vi "Main7.vi"() -> ()   [LabVIEW 2017]
uses:
  <vilib>/Analysis/2dsp.llb/Real FFT.vi
  <vilib>/Analysis/NI_AALPro.lvlib
  atmcd32d.dll
panel:
  in  "index (row)":i32
  out "Angle Integrated Spectrum 2":T1(graph)
  in  "Area Parameteres":T2={"Center angle (deg)"=90.0, "Arc length (deg)"=90.0, "Angle step (deg)"=10.0, "Outer radius "=0.7640449438202247, "Inner radius "=0.0, "Radius"=0.0, "Radial step "=0.5}
  in  "Tab Control":T3(tab)
  out "Current angle":dbl
  in  "Exposure time [ms]":u32=100
  out "Count":i32
  in  "Integration time [s]":dbl=1.0
  out "Ready":bool
  out "Connected":bool
  out "Device":refnum<visa-resource-name>
  in  "Exit":bool
  in  "Take image":bool
  in  "Spectrum":T4(tab)
  out "Fully Integrated Spectrum":dbl(graph)
  out "Angular distribution":dbl[][](graph)
  out "Angle Integrated Spectrum":T5(graph)
  out "Angular distribution 2":dbl[][](graph)
  in  "Energy/Radius":enum32{"Radius", "Energy"}(radio)
  out "Spectrogram up":dbl[][](graph)=[[0.0010313840536425023, 0.0010313840536425023, 0.0010274759814052766, 0.0010401531177745159, 0.00104452387932524, 0.0010522711712232782, 0.001047206375702307, 0.0010453914217880493, 0.0010393489196820073, 0.0010272942106035452, 0.0010408196107141979, 0.0010468510964080136, 0.001062026204249532, 0.001106433361933133, 0.001154520001300267, 0.0011934960677563772, 0.001214033414248973, 0.0012241024150236718, 0.0012391453259184763, 0.0012555680424446059, 0.0012925281054633312, 0.001352528994653044, 0.0014089853532089937, 0.0014660421062312687, 0.0015363130457188075, 0.0015691474623588406, 0.0016108363203256395, 0.0016140062929437132, 0.0015863330654316305, 0.001566139981821102, 0.0015480455247396548, 0.0015630250912641588, 0.0016089194645982896, 0.0016388896140595243, 0.0016752961023638853, 0.001688323009821305, 0.0016919033437948032, 0.0017147706614732288, 0.0017464097973867246, 0.001779717919752482, 0.001837171263614898, 0.00188523587015758, 0.001909243386501412, 0.0019293676175355272, 0.0019505631946586353, 0.0019533283141273984, 0.001977616748982997, 0.0019911972311547808, 0.002017708227177005, 0.002053718124641225, 0.0020883013967221585, 0.002112669700566397, 0.0021315656016372966, 0.0021208218456137463, 0.002105299720787104, 0.002099830072116822, 0.0021012126318512036, 0.0020908214010188896, 0.002095054457416787, 0.002100080695494967, 0.0021084586769929523, 0.0020993728910094368, 0.002104955457905037, 0.0020792872174181134, 0.0020928346503532183, 0.0020942117018814864, 0.002102964241395161, 0.0021093372358679877, 0.002121036665652156, 0.002136567052787968, 0.002154127213876447, 0.002169360157882152, 0.0021869395976920275, 0.0021825908689657556, 0.002171045668952753, 0.0021674267775364637, 0.0021489908116760054, 0.002157660728097984, 0.002145658346977596, 0.002135917084466625, 0.00209696855904108, 0.0020850653256307278, 0.0020535996982097935, 0.002049595232365589, 0.0020524236962046524, 0.0020767176392663643, 0.002111884781195284, 0.002137809153266466, 0.0021668842192343256, 0.00216397037820051, 0.0021656008072099796, 0.0021352698702483386, 0.0021013916485498785, 0.0020823029602650214, 0.0020479290000163844, 0.0020333460243320213, 0.0020002169186649392, 0.0019659586307446764, 0.0019358700548520106, 0.0019274369912928948, 0.0019173046461478957, 0.001900014387158957, 0.0018599917615413628, 0.001814549061108504, 0.0017608991335671654, 0.0017321325271416374, 0.0017011240808280886, 0.0016809695546603515, 0.0016804848325224012, 0.001677022924980334, 0.0016912533754734602, 0.0016999535870290603, 0.0017145172839920274, 0.001701024933118053, 0.0017087557003977521, 0.0017038864461937952, 0.0017154509249281934, 0.0017378638156022909, 0.001773105318313737, 0.0017971238510697952, 0.001824766783448256, 0.0018273914436611356, 0.0018233456662710829, 0.001811169776658133, 0.001808649772361402, 0.0017980740166243004, 0.0017838545825434003, 0.001763256645783561, 0.0017210445082360198, 0.001701132343137258, 0.0016754062664861471, 0.001664623953019805, 0.0016487024832499652, 0.0016273141189128994, 0.0016010950578146683, 0.0015728930425157306, 0.0015352912734848325, 0.0015149109108664593, 0.001483448037548582, 0.0014523514599372237, 0.0014315579818603703, 0.0014274984339550348, 0.0014181675327994876, 0.0014143999198181453, 0.0014053113797315735, 0.0013993515007172275, 0.001408693418285001, 0.0013985390403155494, 0.001397974449188959, 0.0013917694550025816, 0.0013787315311329358, 0.0013626448151797038, 0.0013449083914956062, 0.0013370509354753064, 0.001325880293477993, 0.0013185543793476045, 0.001294420174263172, 0.00127875483607759, 0.0012659041912157889, 0.0012433398248735822, 0.001228894554342046, 0.0012003400138518715, 0.001183988904005212, 0.0011747543964566436, 0.0011585547622780935, 0.0011605046672421217, 0.0011473565792502146, 0.0011370039058606926, 0.0011340652778993677, 0.0011226770617605876, 0.0011216442731143861, 0.0011107600578349525, 0.0011026409620242816, 0.0010866919512238764, 0.0010731362559796018, 0.001051089661012024, 0.0010301832647098524, 0.001009888279286232, 0.0009965887156262153, 0.0009909235256389188, 0.0009767536654130364, 0.0009747817276245561, 0.0009568910741692924, 0.000949947980363763, 0.000956703795161448, 0.0009593917997446279, 0.0009746082191319944, 0.0009815127554947322, 0.0009862085012061277, 0.0009848589907084247, 0.0009587748806599638, 0.0009397330121270677, 0.0009244532483694009, 0.0009160174307072283, 0.0009138141482619988, 0.0009141501488348964, 0.0009184162544694721, 0.0009130457535092251, 0.000912208506180038, 0.0009004897976744733, 0.0008954966088329721, 0.000888658170943591, 0.000878327530378521, 0.0008779392018475493, 0.0008724833236925496, 0.0008753007711193868, 0.0008733894235981503, 0.0008842763929806406, 0.0008803270091975667, 0.0008834474079606231, 0.0008812331091031674, 0.0008784927765619131, 0.0008838109495640858, 0.0008909550928927427, 0.000899184352825675, 0.0009081654828930417, 0.000914194214483801, 0.0009259542345352136, 0.0009387635678511666, 0.0009425339349355657, 0.0009425063939050002, 0.0009326494590656548, 0.0009267529244216092, 0.0009192645182108854, 0.0009126023429171226, 0.0009054058716303917, 0.0008956756255316468, 0.0008975015958581308, 0.0008902445343041561, 0.0008840973762819658, 0.0008824283898297043, 0.0008799772381093866, 0.000884678492026895, 0.0008933897199947213, 0.0008983829088362226, 0.000893860671617389, 0.0008973749071175302, 0.0009013435696219998, 0.0009055848883290665, 0.0009138995254567515, 0.0009202174378684471, 0.000930589389979365, 0.000922150818214136, 0.0009280666315795773, 0.0009267253833910438, 0.0009243623629685353, 0.0009317653919845064, 0.0009418922289233926, 0.0009494384712983037, 0.0009643051195974898, 0.0009718458537662879, 0.0009862966325039368, 0.0009917001827008621, 0.0009979795376697665, 0.001014038712592433, 0.0010172830459930335, 0.0010330585483008768, 0.0010469640146333317, 0.001060098332109956, 0.0010826544361429932, 0.0011030761103072145, 0.0011350760337211167, 0.0011531154087414334, 0.0011576624328877758, 0.0011768364983673857, 0.0011841624124977737, 0.0011999406689086737, 0.0012165093528967996, 0.0012281895039595726, 0.0012561601746017613, 0.0012707651831105765, 0.001307240523991351, 0.001333627585376031, 0.0013666217399933432, 0.0014024911782016796, 0.0014332324765187446, 0.0014678102403935655, 0.0014988241949132272, 0.0015329365153714935, 0.0015343879276822883, 0.0015720971067323913, 0.0016118636007657278, 0.001651087536496926, 0.0016970920739533186, 0.001745473402347502, 0.0017665615694514051, 0.0018051024876245825, 0.0018256783915599696, 0.0018815618966801597, 0.0018972630382054765, 0.0019475088943689358, 0.001967589059754146, 0.0019944801219981727, 0.0020293085092511383, 0.0020797967264835726, 0.002127649267090901, 0.002177592171918141, 0.002209096356781867, 0.0022576126362258207, 0.0022860239633570555, 0.002367479315357191, 0.00239798651491445, 0.002459918030346795, 0.002492961758819125, 0.0025305745442622493, 0.0025619850896220525, 0.0025918974029190997, 0.0026126908809959533, 0.0026649499864937407, 0.002671884817990101, 0.0027487573425041584, 0.0027664331759210126, 0.0028080311484869457, 0.002835572179052315, 0.002897776350687257, 0.0029281981730497637, 0.0029626547563900967, 0.002993387792397992, 0.0030170785868903222, 0.0030149964849795806, 0.0030319039236436605, 0.0030360240618162396, 0.0030334957952103388, 0.0030378693108641195, 0.003026379192912247, 0.0030242502712495446, 0.0030348563221202682, 0.0030418489897808152, 0.0030719182869520852, 0.0030982750532031434, 0.0030908086798168716, 0.0031010319103627363, 0.0031036813575031253, 0.0030762670156783568, 0.003066933360419753, 0.003042223547796504, 0.0030263378813663996, 0.003004663090311454, 0.0029920548065186284, 0.0029706664421815625, 0.0029578268137319874, 0.0029413352446294445, 0.0029132489016588815, 0.0028961762168114094, 0.002857943758180564, 0.00283680050901553, 0.0028030104186148787, 0.0027938640423641197, 0.0027516161014768444, 0.002719478472910115, 0.0026733913123620267, 0.002627637398283779, 0.0025728335015617514, 0.0025436510255746865, 0.002504355483164018, 0.0024615594757684913, 0.002436053727361903, 0.0024182842544411267, 0.0024007185851465346, 0.0023905779776923655, 0.0023550968680150007, 0.002333292634116398, 0.002292746728918062, 0.0022553735504408563, 0.0022384468330553806, 0.002203128215458351, 0.00217902430550754, 0.002143711196116624, 0.0021122262899742946, 0.0020506142504965077, 0.00203825383597877, 0.0020262487007553258, 0.0020074629638066875, 0.0019932738248594093, 0.0019544327094530695, 0.0019488088310116213, 0.0019049882972790627, 0.0018915620448784454, 0.0018528393559035367, 0.001821197465886984, 0.0017890212798774634, 0.0017354539754278208, 0.0016897689139259869, 0.001663423164087155, 0.0016456371665480398, 0.0016412085688331283, 0.001628644350689207, 0.0016130809143167168, 0.0016073331012377244, 0.001603339651805746, 0.0015941712427305346, 0.001588935692820058, 0.0015824029603699523, 0.00157714813173808, 0.0015643332902160138, 0.0015630746651191763, 0.0015527274999357675, 0.0015555421932595482, 0.0015637163711313498, 0.0015732180266764021, 0.001592557338339404, 0.001584653062567143, 0.0015960522951181493, 0.0016165015103129358, 0.0016268707083207973, 0.0016398039762742945, 0.001641899848700319, 0.0016484215647381982, 0.0016487190078683044, 0.0016555629539637985, 0.0016557612493838694, 0.0016741145921526312, 0.0017004658501975761, 0.0017330110860166727, 0.0017605190673453631, 0.0017664348807108045, 0.0017779084740443371, 0.001790398331405732, 0.0018131775177863488, 0.0018366452299310996, 0.0018605453362557267, 0.0018882543671075445, 0.0018984252696953353, 0.001914192509694009, 0.0019416316384462862, 0.0019781785860065308, 0.0020108477564631713, 0.0020298097560074277, 0.0020661143424986973, 0.002068810609391047, 0.002110609631480107, 0.002115869968318093, 0.0021256800834054774, 0.0021556667574850513, 0.002178443189762611, 0.0021840174943490416, 0.002213334921385877, 0.002212183706308245, 0.00223874152208243, 0.0022391546375409104, 0.002258397555596934, 0.0022739802706908193, 0.0023094503639559585, 0.002319709397841558, 0.002351866305129683, 0.002368812301236555, 0.0023749456887434623, 0.002389630566240917, 0.0023986777947816403, 0.00241149814450982, 0.0024190003212358263, 0.0024229882624616918, 0.002422095933071374, 0.002423731870286957, 0.0024201625527256847, 0.0024417767535133868, 0.0024415812121963724, 0.002455808908586442, 0.002457513698378438, 0.0024465385976981386, 0.0024522313287160006, 0.0024169705472831585, 0.0024148361174143426, 0.0023995701241719585, 0.0023793853028705996, 0.0023548297200185167, 0.002332361747283289, 0.0023205108418310103, 0.0022940521737668603, 0.0022523164960481005, 0.0022274744864781374, 0.0022039158889325208, 0.0021684926154193433, 0.0021411526343771015, 0.002118635087786856, 0.002083801192327777, 0.002047124801923875, 0.0020278653592495127, 0.0019697703093749233, 0.0019519264756716211, 0.0019212622922401392, 0.0018812286502103187, 0.0018427428140982722, 0.001812265909674635, 0.00175640994558501, 0.0017214080498394828, 0.0016736711815605288, 0.0016349457384825634, 0.0015946835058990505, 0.0015675610989982752, 0.0015259052902681545, 0.0014996366553149056, 0.001476708747369236, 0.001439175830914751, 0.0014011692087345419, 0.0013630882257718063, 0.0013162216540587178, 0.0012905451512626243, 0.0012539458757443056, 0.0012235736272368167, 0.0012001196856073486, 0.001185272316029558, 0.0011544346241055146, 0.0011379100057662933, 0.0010844501113358553, 0.0010647610285846733, 0.0010130802847287583, 0.0009929670701068693, 0.0009656849252288149, 0.0009476042386626501, 0.0009280005331062204, 0.0009123489654359212, 0.0008921173243826012, 0.0008740696870531149, 0.000861342976828858, 0.0008399518583887359, 0.0008269304591374295, 0.000805963472568014, 0.0007840931401960546, 0.0007730684656607372, 0.0007618757908389714, 0.000755502796366145, 0.0007484440302322409, 0.0007361304354664644, 0.0007236515945172958, 0.0007035631668229157, 0.0006909796699575985, 0.0006775396470416985, 0.0006603843391025302, 0.0006506954045496334, 0.0006404831904159946, 0.0006315406177914192, 0.000626814576946402, 0.0006201799426832045, 0.0006156053775062967, 0.0006078663479174281, 0.0005998298751984535, 0.0005900335306263518, 0.0005812644664943382, 0.0005748804556092857, 0.0005698349388097101, 0.000566761359798615, 0.0005616442363195694, 0.0005622749259195163, 0.0005532993040582626, 0.0005422911541412846, 0.0005348495676825219, 0.0005325361211150309, 0.0005320376284617976, 0.0005307018884793774, 0.0005264054877111798, 0.0005264054877111798, 0.0005228637111804734, 0.0005181238998201733, 0.0005176309153730532, 0.0005136154331166225, 0.0005124091359778592, 0.0005101562796776121, 0.0005055431570579128, 0.0004995529829099451, 0.0004920150028442035, 0.0004884759804165536, 0.00048560345092858563, 0.000481450263519328, 0.000479029406932632, 0.00047415189041950524, 0.00047243608421528277, 0.0004715299843096821, 0.00047353772543789753, 0.00047000971942247376, 0.0004698554896513077, 0.0004721276246729506, 0.0004682388311571205, 0.0004696351614067847, 0.0004644106279085342, 0.00046173088563452376, 0.0004594807834373332, 0.0004550053659704607, 0.0004509155229315034, 0.00044808430498938354, 0.0004430277717775818, 0.0004410696045043841, 0.00043787759906185783, 0.00043347929648056836, 0.0004299017166101269, 0.00042542354504019795, 0.00042215993291820175, 0.00041868425486085215, 0.000416883071461877, 0.0004110388647759057, 0.0004118981449295452, 0.00040788541677617095, 0.00040867033614728403, 0.00040761000647051725, 0.0004041866563712419, 0.00040178507850594175, 0.00039903372955246133, 0.0003977007436730975, 0.0003977310388067194, 0.00039884645054461687, 0.00039690480788975835, 0.000394671230310907, 0.0003933712936682215, 0.00039117076532604856, 0.0003899947633209073, 0.00038895095826247983, 0.00038990112381698505, 0.00038822662915861066, 0.0003852577060636639, 0.00038354740806555447, 0.0003831673418437523, 0.00038108523993301045, 0.00038199133983861106, 0.0003807712721845652, 0.0003789921216100424, 0.0003772350038599718, 0.00037759028315426514, 0.0003756155912627282, 0.0003736216206497954, 0.000373136898511845, 0.0003710079768491419, 0.0003707132878220925, 0.0003699917128212798, 0.00036924259678990177, 0.0003697686304737003, 0.000369484957858877, 0.0003692976788510325, 0.00037006056539769325, 0.00036974108944313496, 0.00036845492331573224, 0.0003671825277036122, 0.0003674441674939832, 0.00036729820003198675, 0.00036671708428705744, 0.0003670723635813507, 0.0003662516408705027, 0.0003653593114801848, 0.0003654336722627113, 0.00036621859163382426, 0.0003649076385789127, 0.0003645000313265452, 0.00036404009611610357, 0.00036481399907499045, 0.00036354435756592694, 0.0003624454704463687, 0.00036318632416857717, 0.000362616224835874, 0.00036201858447260554, 0.0003629026515537539, 0.00036316429134412485, 0.0003618092726403087, 0.00036178173160974337, 0.0003609059268377646, 0.0003606580575626763, 0.00035972441662651027, 0.00035978776099681063, 0.0003598290725426587, 0.0003593278257863689, 0.00035902487445014993, 0.0003587962838964574, 0.00035836939792269413, 0.00035583837721373673, 0.0003554059830338604, 0.0003547532606094612, 0.0003549102444836838, 0.00035429057129596295, 0.0003543126041204152, 0.0003549185067928534, 0.0003548248672889311, 0.00035513057272820676, 0.0003544998831282598, 0.00035434014515098067, 0.000354516407746599, 0.00035333489753534467, 0.0003535855209134895, 0.0003530154215807864, 0.0003527152243476239, 0.0003532798154742139, 0.00035263260125592777, 0.0003519964034498677, 0.000351608074918896, 0.00035093882787615757, 0.000349443349916458, 0.00034942957940117537, 0.0003491624314046913, 0.00034956453045094566, 0.00034901095573658175, 0.00034910184113744744, 0.0003489310867479422, 0.0003488181685226241, 0.0003479836752964935, 0.0003476917403725006, 0.00034843259409470895, 0.0003489586277785075, 0.0003480910853156984, 0.0003474548875096384, 0.0003469619030625183, 0.00034665344352018617, 0.0003463918037298151, 0.00034654052529486815, 0.00034605304905386115, 0.0003454196053508576, 0.00034516347376659963, 0.00034559862204953256, 0.0003448357355028718, 0.0003449403914190202, 0.00034430419361296017, 0.00034424635744877293, 0.000344852260121211, 0.0003448384896059283, 0.0003451028834993559, 0.0003437423565894266, 0.0003425580922751158, 0.00034259664971790727, 0.0003416354677511759, 0.00034174838597649394, 0.00034173461546121124, 0.0003417869434192854, 0.0003409965158420593, 0.00034094143378092864, 0.0003408477942770064, 0.0003402501539137379, 0.0003404980231888262, 0.0003398783500011054, 0.00033904936498108774, 0.00033842969179336696, 0.00033828372433137053, 0.0003380661501899041, 0.00033740791955939176, 0.000338358085113897, 0.0003377081167925543, 0.00033727847671573453, 0.000337388640837996, 0.00033701959102842003, 0.00033749605085720095, 0.00033774116602923275, 0.0003364384752834908, 0.000335931720321088, 0.0003357031297673954, 0.00033592070390886183, 0.0003353395881639325, 0.00033492922680850853, 0.00033513303043469225, 0.00033468961984258985, 0.0003348713906443213, 0.00033494024322073466, 0.0003348108003770775, 0.00033487689885043436, 0.00033441145543387964, 0.0003341993894985263, 0.0003345464064836499, 0.00033424896335354395, 0.00033390194636842026, 0.00033334837165405635, 0.00033337040447850867, 0.0003331583385431553, 0.0003329132233711235, 0.0003332326993256818, 0.0003335301424557878, 0.0003335026014252224, 0.00033401761869679484, 0.0003333428634479433, 0.00033282509207331433, 0.00033313630571870306, 0.0003330839777606288, 0.00033270666564188324, 0.00033214758272140626, 0.00033204843501137094, 0.00033124974512497527, 0.0003311781384455053, 0.00033189695934326144, 0.0003313213518044452, 0.0003320980088663886, 0.0003318336149729611, 0.00033207873014499283, 0.0003325304030462649, 0.0003314094831022544, 0.00033175650008737803]]
  out "Range scan":dbl[][](graph)
  out "Spectrogram down":dbl[][](graph)=[[0.0010313840536425023, 0.0010313840536425023, 0.0010274759814052766, 0.0010401531177745159, 0.00104452387932524, 0.0010522711712232782, 0.001047206375702307, 0.0010453914217880493, 0.0010393489196820073, 0.0010272942106035452, 0.0010408196107141979, 0.0010468510964080136, 0.001062026204249532, 0.001106433361933133, 0.001154520001300267, 0.0011934960677563772, 0.001214033414248973, 0.0012241024150236718, 0.0012391453259184763, 0.0012555680424446059, 0.0012925281054633312, 0.001352528994653044, 0.0014089853532089937, 0.0014660421062312687, 0.0015363130457188075, 0.0015691474623588406, 0.0016108363203256395, 0.0016140062929437132, 0.0015863330654316305, 0.001566139981821102, 0.0015480455247396548, 0.0015630250912641588, 0.0016089194645982896, 0.0016388896140595243, 0.0016752961023638853, 0.001688323009821305, 0.0016919033437948032, 0.0017147706614732288, 0.0017464097973867246, 0.001779717919752482, 0.001837171263614898, 0.00188523587015758, 0.001909243386501412, 0.0019293676175355272, 0.0019505631946586353, 0.0019533283141273984, 0.001977616748982997, 0.0019911972311547808, 0.002017708227177005, 0.002053718124641225, 0.0020883013967221585, 0.002112669700566397, 0.0021315656016372966, 0.0021208218456137463, 0.002105299720787104, 0.002099830072116822, 0.0021012126318512036, 0.0020908214010188896, 0.002095054457416787, 0.002100080695494967, 0.0021084586769929523, 0.0020993728910094368, 0.002104955457905037, 0.0020792872174181134, 0.0020928346503532183, 0.0020942117018814864, 0.002102964241395161, 0.0021093372358679877, 0.002121036665652156, 0.002136567052787968, 0.002154127213876447, 0.002169360157882152, 0.0021869395976920275, 0.0021825908689657556, 0.002171045668952753, 0.0021674267775364637, 0.0021489908116760054, 0.002157660728097984, 0.002145658346977596, 0.002135917084466625, 0.00209696855904108, 0.0020850653256307278, 0.0020535996982097935, 0.002049595232365589, 0.0020524236962046524, 0.0020767176392663643, 0.002111884781195284, 0.002137809153266466, 0.0021668842192343256, 0.00216397037820051, 0.0021656008072099796, 0.0021352698702483386, 0.0021013916485498785, 0.0020823029602650214, 0.0020479290000163844, 0.0020333460243320213, 0.0020002169186649392, 0.0019659586307446764, 0.0019358700548520106, 0.0019274369912928948, 0.0019173046461478957, 0.001900014387158957, 0.0018599917615413628, 0.001814549061108504, 0.0017608991335671654, 0.0017321325271416374, 0.0017011240808280886, 0.0016809695546603515, 0.0016804848325224012, 0.001677022924980334, 0.0016912533754734602, 0.0016999535870290603, 0.0017145172839920274, 0.001701024933118053, 0.0017087557003977521, 0.0017038864461937952, 0.0017154509249281934, 0.0017378638156022909, 0.001773105318313737, 0.0017971238510697952, 0.001824766783448256, 0.0018273914436611356, 0.0018233456662710829, 0.001811169776658133, 0.001808649772361402, 0.0017980740166243004, 0.0017838545825434003, 0.001763256645783561, 0.0017210445082360198, 0.001701132343137258, 0.0016754062664861471, 0.001664623953019805, 0.0016487024832499652, 0.0016273141189128994, 0.0016010950578146683, 0.0015728930425157306, 0.0015352912734848325, 0.0015149109108664593, 0.001483448037548582, 0.0014523514599372237, 0.0014315579818603703, 0.0014274984339550348, 0.0014181675327994876, 0.0014143999198181453, 0.0014053113797315735, 0.0013993515007172275, 0.001408693418285001, 0.0013985390403155494, 0.001397974449188959, 0.0013917694550025816, 0.0013787315311329358, 0.0013626448151797038, 0.0013449083914956062, 0.0013370509354753064, 0.001325880293477993, 0.0013185543793476045, 0.001294420174263172, 0.00127875483607759, 0.0012659041912157889, 0.0012433398248735822, 0.001228894554342046, 0.0012003400138518715, 0.001183988904005212, 0.0011747543964566436, 0.0011585547622780935, 0.0011605046672421217, 0.0011473565792502146, 0.0011370039058606926, 0.0011340652778993677, 0.0011226770617605876, 0.0011216442731143861, 0.0011107600578349525, 0.0011026409620242816, 0.0010866919512238764, 0.0010731362559796018, 0.001051089661012024, 0.0010301832647098524, 0.001009888279286232, 0.0009965887156262153, 0.0009909235256389188, 0.0009767536654130364, 0.0009747817276245561, 0.0009568910741692924, 0.000949947980363763, 0.000956703795161448, 0.0009593917997446279, 0.0009746082191319944, 0.0009815127554947322, 0.0009862085012061277, 0.0009848589907084247, 0.0009587748806599638, 0.0009397330121270677, 0.0009244532483694009, 0.0009160174307072283, 0.0009138141482619988, 0.0009141501488348964, 0.0009184162544694721, 0.0009130457535092251, 0.000912208506180038, 0.0009004897976744733, 0.0008954966088329721, 0.000888658170943591, 0.000878327530378521, 0.0008779392018475493, 0.0008724833236925496, 0.0008753007711193868, 0.0008733894235981503, 0.0008842763929806406, 0.0008803270091975667, 0.0008834474079606231, 0.0008812331091031674, 0.0008784927765619131, 0.0008838109495640858, 0.0008909550928927427, 0.000899184352825675, 0.0009081654828930417, 0.000914194214483801, 0.0009259542345352136, 0.0009387635678511666, 0.0009425339349355657, 0.0009425063939050002, 0.0009326494590656548, 0.0009267529244216092, 0.0009192645182108854, 0.0009126023429171226, 0.0009054058716303917, 0.0008956756255316468, 0.0008975015958581308, 0.0008902445343041561, 0.0008840973762819658, 0.0008824283898297043, 0.0008799772381093866, 0.000884678492026895, 0.0008933897199947213, 0.0008983829088362226, 0.000893860671617389, 0.0008973749071175302, 0.0009013435696219998, 0.0009055848883290665, 0.0009138995254567515, 0.0009202174378684471, 0.000930589389979365, 0.000922150818214136, 0.0009280666315795773, 0.0009267253833910438, 0.0009243623629685353, 0.0009317653919845064, 0.0009418922289233926, 0.0009494384712983037, 0.0009643051195974898, 0.0009718458537662879, 0.0009862966325039368, 0.0009917001827008621, 0.0009979795376697665, 0.001014038712592433, 0.0010172830459930335, 0.0010330585483008768, 0.0010469640146333317, 0.001060098332109956, 0.0010826544361429932, 0.0011030761103072145, 0.0011350760337211167, 0.0011531154087414334, 0.0011576624328877758, 0.0011768364983673857, 0.0011841624124977737, 0.0011999406689086737, 0.0012165093528967996, 0.0012281895039595726, 0.0012561601746017613, 0.0012707651831105765, 0.001307240523991351, 0.001333627585376031, 0.0013666217399933432, 0.0014024911782016796, 0.0014332324765187446, 0.0014678102403935655, 0.0014988241949132272, 0.0015329365153714935, 0.0015343879276822883, 0.0015720971067323913, 0.0016118636007657278, 0.001651087536496926, 0.0016970920739533186, 0.001745473402347502, 0.0017665615694514051, 0.0018051024876245825, 0.0018256783915599696, 0.0018815618966801597, 0.0018972630382054765, 0.0019475088943689358, 0.001967589059754146, 0.0019944801219981727, 0.0020293085092511383, 0.0020797967264835726, 0.002127649267090901, 0.002177592171918141, 0.002209096356781867, 0.0022576126362258207, 0.0022860239633570555, 0.002367479315357191, 0.00239798651491445, 0.002459918030346795, 0.002492961758819125, 0.0025305745442622493, 0.0025619850896220525, 0.0025918974029190997, 0.0026126908809959533, 0.0026649499864937407, 0.002671884817990101, 0.0027487573425041584, 0.0027664331759210126, 0.0028080311484869457, 0.002835572179052315, 0.002897776350687257, 0.0029281981730497637, 0.0029626547563900967, 0.002993387792397992, 0.0030170785868903222, 0.0030149964849795806, 0.0030319039236436605, 0.0030360240618162396, 0.0030334957952103388, 0.0030378693108641195, 0.003026379192912247, 0.0030242502712495446, 0.0030348563221202682, 0.0030418489897808152, 0.0030719182869520852, 0.0030982750532031434, 0.0030908086798168716, 0.0031010319103627363, 0.0031036813575031253, 0.0030762670156783568, 0.003066933360419753, 0.003042223547796504, 0.0030263378813663996, 0.003004663090311454, 0.0029920548065186284, 0.0029706664421815625, 0.0029578268137319874, 0.0029413352446294445, 0.0029132489016588815, 0.0028961762168114094, 0.002857943758180564, 0.00283680050901553, 0.0028030104186148787, 0.0027938640423641197, 0.0027516161014768444, 0.002719478472910115, 0.0026733913123620267, 0.002627637398283779, 0.0025728335015617514, 0.0025436510255746865, 0.002504355483164018, 0.0024615594757684913, 0.002436053727361903, 0.0024182842544411267, 0.0024007185851465346, 0.0023905779776923655, 0.0023550968680150007, 0.002333292634116398, 0.002292746728918062, 0.0022553735504408563, 0.0022384468330553806, 0.002203128215458351, 0.00217902430550754, 0.002143711196116624, 0.0021122262899742946, 0.0020506142504965077, 0.00203825383597877, 0.0020262487007553258, 0.0020074629638066875, 0.0019932738248594093, 0.0019544327094530695, 0.0019488088310116213, 0.0019049882972790627, 0.0018915620448784454, 0.0018528393559035367, 0.001821197465886984, 0.0017890212798774634, 0.0017354539754278208, 0.0016897689139259869, 0.001663423164087155, 0.0016456371665480398, 0.0016412085688331283, 0.001628644350689207, 0.0016130809143167168, 0.0016073331012377244, 0.001603339651805746, 0.0015941712427305346, 0.001588935692820058, 0.0015824029603699523, 0.00157714813173808, 0.0015643332902160138, 0.0015630746651191763, 0.0015527274999357675, 0.0015555421932595482, 0.0015637163711313498, 0.0015732180266764021, 0.001592557338339404, 0.001584653062567143, 0.0015960522951181493, 0.0016165015103129358, 0.0016268707083207973, 0.0016398039762742945, 0.001641899848700319, 0.0016484215647381982, 0.0016487190078683044, 0.0016555629539637985, 0.0016557612493838694, 0.0016741145921526312, 0.0017004658501975761, 0.0017330110860166727, 0.0017605190673453631, 0.0017664348807108045, 0.0017779084740443371, 0.001790398331405732, 0.0018131775177863488, 0.0018366452299310996, 0.0018605453362557267, 0.0018882543671075445, 0.0018984252696953353, 0.001914192509694009, 0.0019416316384462862, 0.0019781785860065308, 0.0020108477564631713, 0.0020298097560074277, 0.0020661143424986973, 0.002068810609391047, 0.002110609631480107, 0.002115869968318093, 0.0021256800834054774, 0.0021556667574850513, 0.002178443189762611, 0.0021840174943490416, 0.002213334921385877, 0.002212183706308245, 0.00223874152208243, 0.0022391546375409104, 0.002258397555596934, 0.0022739802706908193, 0.0023094503639559585, 0.002319709397841558, 0.002351866305129683, 0.002368812301236555, 0.0023749456887434623, 0.002389630566240917, 0.0023986777947816403, 0.00241149814450982, 0.0024190003212358263, 0.0024229882624616918, 0.002422095933071374, 0.002423731870286957, 0.0024201625527256847, 0.0024417767535133868, 0.0024415812121963724, 0.002455808908586442, 0.002457513698378438, 0.0024465385976981386, 0.0024522313287160006, 0.0024169705472831585, 0.0024148361174143426, 0.0023995701241719585, 0.0023793853028705996, 0.0023548297200185167, 0.002332361747283289, 0.0023205108418310103, 0.0022940521737668603, 0.0022523164960481005, 0.0022274744864781374, 0.0022039158889325208, 0.0021684926154193433, 0.0021411526343771015, 0.002118635087786856, 0.002083801192327777, 0.002047124801923875, 0.0020278653592495127, 0.0019697703093749233, 0.0019519264756716211, 0.0019212622922401392, 0.0018812286502103187, 0.0018427428140982722, 0.001812265909674635, 0.00175640994558501, 0.0017214080498394828, 0.0016736711815605288, 0.0016349457384825634, 0.0015946835058990505, 0.0015675610989982752, 0.0015259052902681545, 0.0014996366553149056, 0.001476708747369236, 0.001439175830914751, 0.0014011692087345419, 0.0013630882257718063, 0.0013162216540587178, 0.0012905451512626243, 0.0012539458757443056, 0.0012235736272368167, 0.0012001196856073486, 0.001185272316029558, 0.0011544346241055146, 0.0011379100057662933, 0.0010844501113358553, 0.0010647610285846733, 0.0010130802847287583, 0.0009929670701068693, 0.0009656849252288149, 0.0009476042386626501, 0.0009280005331062204, 0.0009123489654359212, 0.0008921173243826012, 0.0008740696870531149, 0.000861342976828858, 0.0008399518583887359, 0.0008269304591374295, 0.000805963472568014, 0.0007840931401960546, 0.0007730684656607372, 0.0007618757908389714, 0.000755502796366145, 0.0007484440302322409, 0.0007361304354664644, 0.0007236515945172958, 0.0007035631668229157, 0.0006909796699575985, 0.0006775396470416985, 0.0006603843391025302, 0.0006506954045496334, 0.0006404831904159946, 0.0006315406177914192, 0.000626814576946402, 0.0006201799426832045, 0.0006156053775062967, 0.0006078663479174281, 0.0005998298751984535, 0.0005900335306263518, 0.0005812644664943382, 0.0005748804556092857, 0.0005698349388097101, 0.000566761359798615, 0.0005616442363195694, 0.0005622749259195163, 0.0005532993040582626, 0.0005422911541412846, 0.0005348495676825219, 0.0005325361211150309, 0.0005320376284617976, 0.0005307018884793774, 0.0005264054877111798, 0.0005264054877111798, 0.0005228637111804734, 0.0005181238998201733, 0.0005176309153730532, 0.0005136154331166225, 0.0005124091359778592, 0.0005101562796776121, 0.0005055431570579128, 0.0004995529829099451, 0.0004920150028442035, 0.0004884759804165536, 0.00048560345092858563, 0.000481450263519328, 0.000479029406932632, 0.00047415189041950524, 0.00047243608421528277, 0.0004715299843096821, 0.00047353772543789753, 0.00047000971942247376, 0.0004698554896513077, 0.0004721276246729506, 0.0004682388311571205, 0.0004696351614067847, 0.0004644106279085342, 0.00046173088563452376, 0.0004594807834373332, 0.0004550053659704607, 0.0004509155229315034, 0.00044808430498938354, 0.0004430277717775818, 0.0004410696045043841, 0.00043787759906185783, 0.00043347929648056836, 0.0004299017166101269, 0.00042542354504019795, 0.00042215993291820175, 0.00041868425486085215, 0.000416883071461877, 0.0004110388647759057, 0.0004118981449295452, 0.00040788541677617095, 0.00040867033614728403, 0.00040761000647051725, 0.0004041866563712419, 0.00040178507850594175, 0.00039903372955246133, 0.0003977007436730975, 0.0003977310388067194, 0.00039884645054461687, 0.00039690480788975835, 0.000394671230310907, 0.0003933712936682215, 0.00039117076532604856, 0.0003899947633209073, 0.00038895095826247983, 0.00038990112381698505, 0.00038822662915861066, 0.0003852577060636639, 0.00038354740806555447, 0.0003831673418437523, 0.00038108523993301045, 0.00038199133983861106, 0.0003807712721845652, 0.0003789921216100424, 0.0003772350038599718, 0.00037759028315426514, 0.0003756155912627282, 0.0003736216206497954, 0.000373136898511845, 0.0003710079768491419, 0.0003707132878220925, 0.0003699917128212798, 0.00036924259678990177, 0.0003697686304737003, 0.000369484957858877, 0.0003692976788510325, 0.00037006056539769325, 0.00036974108944313496, 0.00036845492331573224, 0.0003671825277036122, 0.0003674441674939832, 0.00036729820003198675, 0.00036671708428705744, 0.0003670723635813507, 0.0003662516408705027, 0.0003653593114801848, 0.0003654336722627113, 0.00036621859163382426, 0.0003649076385789127, 0.0003645000313265452, 0.00036404009611610357, 0.00036481399907499045, 0.00036354435756592694, 0.0003624454704463687, 0.00036318632416857717, 0.000362616224835874, 0.00036201858447260554, 0.0003629026515537539, 0.00036316429134412485, 0.0003618092726403087, 0.00036178173160974337, 0.0003609059268377646, 0.0003606580575626763, 0.00035972441662651027, 0.00035978776099681063, 0.0003598290725426587, 0.0003593278257863689, 0.00035902487445014993, 0.0003587962838964574, 0.00035836939792269413, 0.00035583837721373673, 0.0003554059830338604, 0.0003547532606094612, 0.0003549102444836838, 0.00035429057129596295, 0.0003543126041204152, 0.0003549185067928534, 0.0003548248672889311, 0.00035513057272820676, 0.0003544998831282598, 0.00035434014515098067, 0.000354516407746599, 0.00035333489753534467, 0.0003535855209134895, 0.0003530154215807864, 0.0003527152243476239, 0.0003532798154742139, 0.00035263260125592777, 0.0003519964034498677, 0.000351608074918896, 0.00035093882787615757, 0.000349443349916458, 0.00034942957940117537, 0.0003491624314046913, 0.00034956453045094566, 0.00034901095573658175, 0.00034910184113744744, 0.0003489310867479422, 0.0003488181685226241, 0.0003479836752964935, 0.0003476917403725006, 0.00034843259409470895, 0.0003489586277785075, 0.0003480910853156984, 0.0003474548875096384, 0.0003469619030625183, 0.00034665344352018617, 0.0003463918037298151, 0.00034654052529486815, 0.00034605304905386115, 0.0003454196053508576, 0.00034516347376659963, 0.00034559862204953256, 0.0003448357355028718, 0.0003449403914190202, 0.00034430419361296017, 0.00034424635744877293, 0.000344852260121211, 0.0003448384896059283, 0.0003451028834993559, 0.0003437423565894266, 0.0003425580922751158, 0.00034259664971790727, 0.0003416354677511759, 0.00034174838597649394, 0.00034173461546121124, 0.0003417869434192854, 0.0003409965158420593, 0.00034094143378092864, 0.0003408477942770064, 0.0003402501539137379, 0.0003404980231888262, 0.0003398783500011054, 0.00033904936498108774, 0.00033842969179336696, 0.00033828372433137053, 0.0003380661501899041, 0.00033740791955939176, 0.000338358085113897, 0.0003377081167925543, 0.00033727847671573453, 0.000337388640837996, 0.00033701959102842003, 0.00033749605085720095, 0.00033774116602923275, 0.0003364384752834908, 0.000335931720321088, 0.0003357031297673954, 0.00033592070390886183, 0.0003353395881639325, 0.00033492922680850853, 0.00033513303043469225, 0.00033468961984258985, 0.0003348713906443213, 0.00033494024322073466, 0.0003348108003770775, 0.00033487689885043436, 0.00033441145543387964, 0.0003341993894985263, 0.0003345464064836499, 0.00033424896335354395, 0.00033390194636842026, 0.00033334837165405635, 0.00033337040447850867, 0.0003331583385431553, 0.0003329132233711235, 0.0003332326993256818, 0.0003335301424557878, 0.0003335026014252224, 0.00033401761869679484, 0.0003333428634479433, 0.00033282509207331433, 0.00033313630571870306, 0.0003330839777606288, 0.00033270666564188324, 0.00033214758272140626, 0.00033204843501137094, 0.00033124974512497527, 0.0003311781384455053, 0.00033189695934326144, 0.0003313213518044452, 0.0003320980088663886, 0.0003318336149729611, 0.00033207873014499283, 0.0003325304030462649, 0.0003314094831022544, 0.00033175650008737803]]
  out "FFT":dbl[](graph)
  out "Asymetry spectrogarm":dbl[][](graph)=[[0.0010313840536425023, 0.0010313840536425023, 0.0010274759814052766, 0.0010401531177745159, 0.00104452387932524, 0.0010522711712232782, 0.001047206375702307, 0.0010453914217880493, 0.0010393489196820073, 0.0010272942106035452, 0.0010408196107141979, 0.0010468510964080136, 0.001062026204249532, 0.001106433361933133, 0.001154520001300267, 0.0011934960677563772, 0.001214033414248973, 0.0012241024150236718, 0.0012391453259184763, 0.0012555680424446059, 0.0012925281054633312, 0.001352528994653044, 0.0014089853532089937, 0.0014660421062312687, 0.0015363130457188075, 0.0015691474623588406, 0.0016108363203256395, 0.0016140062929437132, 0.0015863330654316305, 0.001566139981821102, 0.0015480455247396548, 0.0015630250912641588, 0.0016089194645982896, 0.0016388896140595243, 0.0016752961023638853, 0.001688323009821305, 0.0016919033437948032, 0.0017147706614732288, 0.0017464097973867246, 0.001779717919752482, 0.001837171263614898, 0.00188523587015758, 0.001909243386501412, 0.0019293676175355272, 0.0019505631946586353, 0.0019533283141273984, 0.001977616748982997, 0.0019911972311547808, 0.002017708227177005, 0.002053718124641225, 0.0020883013967221585, 0.002112669700566397, 0.0021315656016372966, 0.0021208218456137463, 0.002105299720787104, 0.002099830072116822, 0.0021012126318512036, 0.0020908214010188896, 0.002095054457416787, 0.002100080695494967, 0.0021084586769929523, 0.0020993728910094368, 0.002104955457905037, 0.0020792872174181134, 0.0020928346503532183, 0.0020942117018814864, 0.002102964241395161, 0.0021093372358679877, 0.002121036665652156, 0.002136567052787968, 0.002154127213876447, 0.002169360157882152, 0.0021869395976920275, 0.0021825908689657556, 0.002171045668952753, 0.0021674267775364637, 0.0021489908116760054, 0.002157660728097984, 0.002145658346977596, 0.002135917084466625, 0.00209696855904108, 0.0020850653256307278, 0.0020535996982097935, 0.002049595232365589, 0.0020524236962046524, 0.0020767176392663643, 0.002111884781195284, 0.002137809153266466, 0.0021668842192343256, 0.00216397037820051, 0.0021656008072099796, 0.0021352698702483386, 0.0021013916485498785, 0.0020823029602650214, 0.0020479290000163844, 0.0020333460243320213, 0.0020002169186649392, 0.0019659586307446764, 0.0019358700548520106, 0.0019274369912928948, 0.0019173046461478957, 0.001900014387158957, 0.0018599917615413628, 0.001814549061108504, 0.0017608991335671654, 0.0017321325271416374, 0.0017011240808280886, 0.0016809695546603515, 0.0016804848325224012, 0.001677022924980334, 0.0016912533754734602, 0.0016999535870290603, 0.0017145172839920274, 0.001701024933118053, 0.0017087557003977521, 0.0017038864461937952, 0.0017154509249281934, 0.0017378638156022909, 0.001773105318313737, 0.0017971238510697952, 0.001824766783448256, 0.0018273914436611356, 0.0018233456662710829, 0.001811169776658133, 0.001808649772361402, 0.0017980740166243004, 0.0017838545825434003, 0.001763256645783561, 0.0017210445082360198, 0.001701132343137258, 0.0016754062664861471, 0.001664623953019805, 0.0016487024832499652, 0.0016273141189128994, 0.0016010950578146683, 0.0015728930425157306, 0.0015352912734848325, 0.0015149109108664593, 0.001483448037548582, 0.0014523514599372237, 0.0014315579818603703, 0.0014274984339550348, 0.0014181675327994876, 0.0014143999198181453, 0.0014053113797315735, 0.0013993515007172275, 0.001408693418285001, 0.0013985390403155494, 0.001397974449188959, 0.0013917694550025816, 0.0013787315311329358, 0.0013626448151797038, 0.0013449083914956062, 0.0013370509354753064, 0.001325880293477993, 0.0013185543793476045, 0.001294420174263172, 0.00127875483607759, 0.0012659041912157889, 0.0012433398248735822, 0.001228894554342046, 0.0012003400138518715, 0.001183988904005212, 0.0011747543964566436, 0.0011585547622780935, 0.0011605046672421217, 0.0011473565792502146, 0.0011370039058606926, 0.0011340652778993677, 0.0011226770617605876, 0.0011216442731143861, 0.0011107600578349525, 0.0011026409620242816, 0.0010866919512238764, 0.0010731362559796018, 0.001051089661012024, 0.0010301832647098524, 0.001009888279286232, 0.0009965887156262153, 0.0009909235256389188, 0.0009767536654130364, 0.0009747817276245561, 0.0009568910741692924, 0.000949947980363763, 0.000956703795161448, 0.0009593917997446279, 0.0009746082191319944, 0.0009815127554947322, 0.0009862085012061277, 0.0009848589907084247, 0.0009587748806599638, 0.0009397330121270677, 0.0009244532483694009, 0.0009160174307072283, 0.0009138141482619988, 0.0009141501488348964, 0.0009184162544694721, 0.0009130457535092251, 0.000912208506180038, 0.0009004897976744733, 0.0008954966088329721, 0.000888658170943591, 0.000878327530378521, 0.0008779392018475493, 0.0008724833236925496, 0.0008753007711193868, 0.0008733894235981503, 0.0008842763929806406, 0.0008803270091975667, 0.0008834474079606231, 0.0008812331091031674, 0.0008784927765619131, 0.0008838109495640858, 0.0008909550928927427, 0.000899184352825675, 0.0009081654828930417, 0.000914194214483801, 0.0009259542345352136, 0.0009387635678511666, 0.0009425339349355657, 0.0009425063939050002, 0.0009326494590656548, 0.0009267529244216092, 0.0009192645182108854, 0.0009126023429171226, 0.0009054058716303917, 0.0008956756255316468, 0.0008975015958581308, 0.0008902445343041561, 0.0008840973762819658, 0.0008824283898297043, 0.0008799772381093866, 0.000884678492026895, 0.0008933897199947213, 0.0008983829088362226, 0.000893860671617389, 0.0008973749071175302, 0.0009013435696219998, 0.0009055848883290665, 0.0009138995254567515, 0.0009202174378684471, 0.000930589389979365, 0.000922150818214136, 0.0009280666315795773, 0.0009267253833910438, 0.0009243623629685353, 0.0009317653919845064, 0.0009418922289233926, 0.0009494384712983037, 0.0009643051195974898, 0.0009718458537662879, 0.0009862966325039368, 0.0009917001827008621, 0.0009979795376697665, 0.001014038712592433, 0.0010172830459930335, 0.0010330585483008768, 0.0010469640146333317, 0.001060098332109956, 0.0010826544361429932, 0.0011030761103072145, 0.0011350760337211167, 0.0011531154087414334, 0.0011576624328877758, 0.0011768364983673857, 0.0011841624124977737, 0.0011999406689086737, 0.0012165093528967996, 0.0012281895039595726, 0.0012561601746017613, 0.0012707651831105765, 0.001307240523991351, 0.001333627585376031, 0.0013666217399933432, 0.0014024911782016796, 0.0014332324765187446, 0.0014678102403935655, 0.0014988241949132272, 0.0015329365153714935, 0.0015343879276822883, 0.0015720971067323913, 0.0016118636007657278, 0.001651087536496926, 0.0016970920739533186, 0.001745473402347502, 0.0017665615694514051, 0.0018051024876245825, 0.0018256783915599696, 0.0018815618966801597, 0.0018972630382054765, 0.0019475088943689358, 0.001967589059754146, 0.0019944801219981727, 0.0020293085092511383, 0.0020797967264835726, 0.002127649267090901, 0.002177592171918141, 0.002209096356781867, 0.0022576126362258207, 0.0022860239633570555, 0.002367479315357191, 0.00239798651491445, 0.002459918030346795, 0.002492961758819125, 0.0025305745442622493, 0.0025619850896220525, 0.0025918974029190997, 0.0026126908809959533, 0.0026649499864937407, 0.002671884817990101, 0.0027487573425041584, 0.0027664331759210126, 0.0028080311484869457, 0.002835572179052315, 0.002897776350687257, 0.0029281981730497637, 0.0029626547563900967, 0.002993387792397992, 0.0030170785868903222, 0.0030149964849795806, 0.0030319039236436605, 0.0030360240618162396, 0.0030334957952103388, 0.0030378693108641195, 0.003026379192912247, 0.0030242502712495446, 0.0030348563221202682, 0.0030418489897808152, 0.0030719182869520852, 0.0030982750532031434, 0.0030908086798168716, 0.0031010319103627363, 0.0031036813575031253, 0.0030762670156783568, 0.003066933360419753, 0.003042223547796504, 0.0030263378813663996, 0.003004663090311454, 0.0029920548065186284, 0.0029706664421815625, 0.0029578268137319874, 0.0029413352446294445, 0.0029132489016588815, 0.0028961762168114094, 0.002857943758180564, 0.00283680050901553, 0.0028030104186148787, 0.0027938640423641197, 0.0027516161014768444, 0.002719478472910115, 0.0026733913123620267, 0.002627637398283779, 0.0025728335015617514, 0.0025436510255746865, 0.002504355483164018, 0.0024615594757684913, 0.002436053727361903, 0.0024182842544411267, 0.0024007185851465346, 0.0023905779776923655, 0.0023550968680150007, 0.002333292634116398, 0.002292746728918062, 0.0022553735504408563, 0.0022384468330553806, 0.002203128215458351, 0.00217902430550754, 0.002143711196116624, 0.0021122262899742946, 0.0020506142504965077, 0.00203825383597877, 0.0020262487007553258, 0.0020074629638066875, 0.0019932738248594093, 0.0019544327094530695, 0.0019488088310116213, 0.0019049882972790627, 0.0018915620448784454, 0.0018528393559035367, 0.001821197465886984, 0.0017890212798774634, 0.0017354539754278208, 0.0016897689139259869, 0.001663423164087155, 0.0016456371665480398, 0.0016412085688331283, 0.001628644350689207, 0.0016130809143167168, 0.0016073331012377244, 0.001603339651805746, 0.0015941712427305346, 0.001588935692820058, 0.0015824029603699523, 0.00157714813173808, 0.0015643332902160138, 0.0015630746651191763, 0.0015527274999357675, 0.0015555421932595482, 0.0015637163711313498, 0.0015732180266764021, 0.001592557338339404, 0.001584653062567143, 0.0015960522951181493, 0.0016165015103129358, 0.0016268707083207973, 0.0016398039762742945, 0.001641899848700319, 0.0016484215647381982, 0.0016487190078683044, 0.0016555629539637985, 0.0016557612493838694, 0.0016741145921526312, 0.0017004658501975761, 0.0017330110860166727, 0.0017605190673453631, 0.0017664348807108045, 0.0017779084740443371, 0.001790398331405732, 0.0018131775177863488, 0.0018366452299310996, 0.0018605453362557267, 0.0018882543671075445, 0.0018984252696953353, 0.001914192509694009, 0.0019416316384462862, 0.0019781785860065308, 0.0020108477564631713, 0.0020298097560074277, 0.0020661143424986973, 0.002068810609391047, 0.002110609631480107, 0.002115869968318093, 0.0021256800834054774, 0.0021556667574850513, 0.002178443189762611, 0.0021840174943490416, 0.002213334921385877, 0.002212183706308245, 0.00223874152208243, 0.0022391546375409104, 0.002258397555596934, 0.0022739802706908193, 0.0023094503639559585, 0.002319709397841558, 0.002351866305129683, 0.002368812301236555, 0.0023749456887434623, 0.002389630566240917, 0.0023986777947816403, 0.00241149814450982, 0.0024190003212358263, 0.0024229882624616918, 0.002422095933071374, 0.002423731870286957, 0.0024201625527256847, 0.0024417767535133868, 0.0024415812121963724, 0.002455808908586442, 0.002457513698378438, 0.0024465385976981386, 0.0024522313287160006, 0.0024169705472831585, 0.0024148361174143426, 0.0023995701241719585, 0.0023793853028705996, 0.0023548297200185167, 0.002332361747283289, 0.0023205108418310103, 0.0022940521737668603, 0.0022523164960481005, 0.0022274744864781374, 0.0022039158889325208, 0.0021684926154193433, 0.0021411526343771015, 0.002118635087786856, 0.002083801192327777, 0.002047124801923875, 0.0020278653592495127, 0.0019697703093749233, 0.0019519264756716211, 0.0019212622922401392, 0.0018812286502103187, 0.0018427428140982722, 0.001812265909674635, 0.00175640994558501, 0.0017214080498394828, 0.0016736711815605288, 0.0016349457384825634, 0.0015946835058990505, 0.0015675610989982752, 0.0015259052902681545, 0.0014996366553149056, 0.001476708747369236, 0.001439175830914751, 0.0014011692087345419, 0.0013630882257718063, 0.0013162216540587178, 0.0012905451512626243, 0.0012539458757443056, 0.0012235736272368167, 0.0012001196856073486, 0.001185272316029558, 0.0011544346241055146, 0.0011379100057662933, 0.0010844501113358553, 0.0010647610285846733, 0.0010130802847287583, 0.0009929670701068693, 0.0009656849252288149, 0.0009476042386626501, 0.0009280005331062204, 0.0009123489654359212, 0.0008921173243826012, 0.0008740696870531149, 0.000861342976828858, 0.0008399518583887359, 0.0008269304591374295, 0.000805963472568014, 0.0007840931401960546, 0.0007730684656607372, 0.0007618757908389714, 0.000755502796366145, 0.0007484440302322409, 0.0007361304354664644, 0.0007236515945172958, 0.0007035631668229157, 0.0006909796699575985, 0.0006775396470416985, 0.0006603843391025302, 0.0006506954045496334, 0.0006404831904159946, 0.0006315406177914192, 0.000626814576946402, 0.0006201799426832045, 0.0006156053775062967, 0.0006078663479174281, 0.0005998298751984535, 0.0005900335306263518, 0.0005812644664943382, 0.0005748804556092857, 0.0005698349388097101, 0.000566761359798615, 0.0005616442363195694, 0.0005622749259195163, 0.0005532993040582626, 0.0005422911541412846, 0.0005348495676825219, 0.0005325361211150309, 0.0005320376284617976, 0.0005307018884793774, 0.0005264054877111798, 0.0005264054877111798, 0.0005228637111804734, 0.0005181238998201733, 0.0005176309153730532, 0.0005136154331166225, 0.0005124091359778592, 0.0005101562796776121, 0.0005055431570579128, 0.0004995529829099451, 0.0004920150028442035, 0.0004884759804165536, 0.00048560345092858563, 0.000481450263519328, 0.000479029406932632, 0.00047415189041950524, 0.00047243608421528277, 0.0004715299843096821, 0.00047353772543789753, 0.00047000971942247376, 0.0004698554896513077, 0.0004721276246729506, 0.0004682388311571205, 0.0004696351614067847, 0.0004644106279085342, 0.00046173088563452376, 0.0004594807834373332, 0.0004550053659704607, 0.0004509155229315034, 0.00044808430498938354, 0.0004430277717775818, 0.0004410696045043841, 0.00043787759906185783, 0.00043347929648056836, 0.0004299017166101269, 0.00042542354504019795, 0.00042215993291820175, 0.00041868425486085215, 0.000416883071461877, 0.0004110388647759057, 0.0004118981449295452, 0.00040788541677617095, 0.00040867033614728403, 0.00040761000647051725, 0.0004041866563712419, 0.00040178507850594175, 0.00039903372955246133, 0.0003977007436730975, 0.0003977310388067194, 0.00039884645054461687, 0.00039690480788975835, 0.000394671230310907, 0.0003933712936682215, 0.00039117076532604856, 0.0003899947633209073, 0.00038895095826247983, 0.00038990112381698505, 0.00038822662915861066, 0.0003852577060636639, 0.00038354740806555447, 0.0003831673418437523, 0.00038108523993301045, 0.00038199133983861106, 0.0003807712721845652, 0.0003789921216100424, 0.0003772350038599718, 0.00037759028315426514, 0.0003756155912627282, 0.0003736216206497954, 0.000373136898511845, 0.0003710079768491419, 0.0003707132878220925, 0.0003699917128212798, 0.00036924259678990177, 0.0003697686304737003, 0.000369484957858877, 0.0003692976788510325, 0.00037006056539769325, 0.00036974108944313496, 0.00036845492331573224, 0.0003671825277036122, 0.0003674441674939832, 0.00036729820003198675, 0.00036671708428705744, 0.0003670723635813507, 0.0003662516408705027, 0.0003653593114801848, 0.0003654336722627113, 0.00036621859163382426, 0.0003649076385789127, 0.0003645000313265452, 0.00036404009611610357, 0.00036481399907499045, 0.00036354435756592694, 0.0003624454704463687, 0.00036318632416857717, 0.000362616224835874, 0.00036201858447260554, 0.0003629026515537539, 0.00036316429134412485, 0.0003618092726403087, 0.00036178173160974337, 0.0003609059268377646, 0.0003606580575626763, 0.00035972441662651027, 0.00035978776099681063, 0.0003598290725426587, 0.0003593278257863689, 0.00035902487445014993, 0.0003587962838964574, 0.00035836939792269413, 0.00035583837721373673, 0.0003554059830338604, 0.0003547532606094612, 0.0003549102444836838, 0.00035429057129596295, 0.0003543126041204152, 0.0003549185067928534, 0.0003548248672889311, 0.00035513057272820676, 0.0003544998831282598, 0.00035434014515098067, 0.000354516407746599, 0.00035333489753534467, 0.0003535855209134895, 0.0003530154215807864, 0.0003527152243476239, 0.0003532798154742139, 0.00035263260125592777, 0.0003519964034498677, 0.000351608074918896, 0.00035093882787615757, 0.000349443349916458, 0.00034942957940117537, 0.0003491624314046913, 0.00034956453045094566, 0.00034901095573658175, 0.00034910184113744744, 0.0003489310867479422, 0.0003488181685226241, 0.0003479836752964935, 0.0003476917403725006, 0.00034843259409470895, 0.0003489586277785075, 0.0003480910853156984, 0.0003474548875096384, 0.0003469619030625183, 0.00034665344352018617, 0.0003463918037298151, 0.00034654052529486815, 0.00034605304905386115, 0.0003454196053508576, 0.00034516347376659963, 0.00034559862204953256, 0.0003448357355028718, 0.0003449403914190202, 0.00034430419361296017, 0.00034424635744877293, 0.000344852260121211, 0.0003448384896059283, 0.0003451028834993559, 0.0003437423565894266, 0.0003425580922751158, 0.00034259664971790727, 0.0003416354677511759, 0.00034174838597649394, 0.00034173461546121124, 0.0003417869434192854, 0.0003409965158420593, 0.00034094143378092864, 0.0003408477942770064, 0.0003402501539137379, 0.0003404980231888262, 0.0003398783500011054, 0.00033904936498108774, 0.00033842969179336696, 0.00033828372433137053, 0.0003380661501899041, 0.00033740791955939176, 0.000338358085113897, 0.0003377081167925543, 0.00033727847671573453, 0.000337388640837996, 0.00033701959102842003, 0.00033749605085720095, 0.00033774116602923275, 0.0003364384752834908, 0.000335931720321088, 0.0003357031297673954, 0.00033592070390886183, 0.0003353395881639325, 0.00033492922680850853, 0.00033513303043469225, 0.00033468961984258985, 0.0003348713906443213, 0.00033494024322073466, 0.0003348108003770775, 0.00033487689885043436, 0.00033441145543387964, 0.0003341993894985263, 0.0003345464064836499, 0.00033424896335354395, 0.00033390194636842026, 0.00033334837165405635, 0.00033337040447850867, 0.0003331583385431553, 0.0003329132233711235, 0.0003332326993256818, 0.0003335301424557878, 0.0003335026014252224, 0.00033401761869679484, 0.0003333428634479433, 0.00033282509207331433, 0.00033313630571870306, 0.0003330839777606288, 0.00033270666564188324, 0.00033214758272140626, 0.00033204843501137094, 0.00033124974512497527, 0.0003311781384455053, 0.00033189695934326144, 0.0003313213518044452, 0.0003320980088663886, 0.0003318336149729611, 0.00033207873014499283, 0.0003325304030462649, 0.0003314094831022544, 0.00033175650008737803]]
  in  "Stop":bool
  out "Picture":cluster{dbl[], dbl[]}[](graph)
  in  "Start Measurement":bool
  out "CCD IMAGE":dbl[][](graph)
  in  "Arc length (deg)":dbl=90.0
  in  "Angle step (deg)":dbl=1.0
  in  "Center angle (deg)":dbl=90.0
  in  "Radial step":dbl=1.0
  in  "Visible":bool=TRUE
  in  "Inner radius":dbl(slide) scale=0.0..1.0
  in  "Outer radius":dbl(slide)=0.9325842696629213 scale=0.0..1.0
  in  "Path":string="E:\\Data\\Data Rabitt\\"
  in  "Name":string="image"
  in  "Index":i32=1
  in  "Run Scan":bool
  in  "Analyze":bool
  in  "Save image":bool
  in  "Start Delay (fs)":dbl format="%.3f"
  out "Current Delay (fs)":dbl
  out "Actual delay  (fs)":dbl=inf format="%.3f"
  in  "Angle":dbl min=0.0 max=5.0 format="%.3f"
  in  "Delay Stage Move":bool
  in  "Step (fs)":dbl=0.13 format="%.3f"
  in  "Max Steps":i32=60
  out "StepNb":i32
  out "Angle [deg]":ext(graph)
  out "Nb of shot":i32
  out "XUV":dbl[][](graph)=[[0.0010313840536425023, 0.0010313840536425023, 0.0010274759814052766, 0.0010401531177745159, 0.00104452387932524, 0.0010522711712232782, 0.001047206375702307, 0.0010453914217880493, 0.0010393489196820073, 0.0010272942106035452, 0.0010408196107141979, 0.0010468510964080136, 0.001062026204249532, 0.001106433361933133, 0.001154520001300267, 0.0011934960677563772, 0.001214033414248973, 0.0012241024150236718, 0.0012391453259184763, 0.0012555680424446059, 0.0012925281054633312, 0.001352528994653044, 0.0014089853532089937, 0.0014660421062312687, 0.0015363130457188075, 0.0015691474623588406, 0.0016108363203256395, 0.0016140062929437132, 0.0015863330654316305, 0.001566139981821102, 0.0015480455247396548, 0.0015630250912641588, 0.0016089194645982896, 0.0016388896140595243, 0.0016752961023638853, 0.001688323009821305, 0.0016919033437948032, 0.0017147706614732288, 0.0017464097973867246, 0.001779717919752482, 0.001837171263614898, 0.00188523587015758, 0.001909243386501412, 0.0019293676175355272, 0.0019505631946586353, 0.0019533283141273984, 0.001977616748982997, 0.0019911972311547808, 0.002017708227177005, 0.002053718124641225, 0.0020883013967221585, 0.002112669700566397, 0.0021315656016372966, 0.0021208218456137463, 0.002105299720787104, 0.002099830072116822, 0.0021012126318512036, 0.0020908214010188896, 0.002095054457416787, 0.002100080695494967, 0.0021084586769929523, 0.0020993728910094368, 0.002104955457905037, 0.0020792872174181134, 0.0020928346503532183, 0.0020942117018814864, 0.002102964241395161, 0.0021093372358679877, 0.002121036665652156, 0.002136567052787968, 0.002154127213876447, 0.002169360157882152, 0.0021869395976920275, 0.0021825908689657556, 0.002171045668952753, 0.0021674267775364637, 0.0021489908116760054, 0.002157660728097984, 0.002145658346977596, 0.002135917084466625, 0.00209696855904108, 0.0020850653256307278, 0.0020535996982097935, 0.002049595232365589, 0.0020524236962046524, 0.0020767176392663643, 0.002111884781195284, 0.002137809153266466, 0.0021668842192343256, 0.00216397037820051, 0.0021656008072099796, 0.0021352698702483386, 0.0021013916485498785, 0.0020823029602650214, 0.0020479290000163844, 0.0020333460243320213, 0.0020002169186649392, 0.0019659586307446764, 0.0019358700548520106, 0.0019274369912928948, 0.0019173046461478957, 0.001900014387158957, 0.0018599917615413628, 0.001814549061108504, 0.0017608991335671654, 0.0017321325271416374, 0.0017011240808280886, 0.0016809695546603515, 0.0016804848325224012, 0.001677022924980334, 0.0016912533754734602, 0.0016999535870290603, 0.0017145172839920274, 0.001701024933118053, 0.0017087557003977521, 0.0017038864461937952, 0.0017154509249281934, 0.0017378638156022909, 0.001773105318313737, 0.0017971238510697952, 0.001824766783448256, 0.0018273914436611356, 0.0018233456662710829, 0.001811169776658133, 0.001808649772361402, 0.0017980740166243004, 0.0017838545825434003, 0.001763256645783561, 0.0017210445082360198, 0.001701132343137258, 0.0016754062664861471, 0.001664623953019805, 0.0016487024832499652, 0.0016273141189128994, 0.0016010950578146683, 0.0015728930425157306, 0.0015352912734848325, 0.0015149109108664593, 0.001483448037548582, 0.0014523514599372237, 0.0014315579818603703, 0.0014274984339550348, 0.0014181675327994876, 0.0014143999198181453, 0.0014053113797315735, 0.0013993515007172275, 0.001408693418285001, 0.0013985390403155494, 0.001397974449188959, 0.0013917694550025816, 0.0013787315311329358, 0.0013626448151797038, 0.0013449083914956062, 0.0013370509354753064, 0.001325880293477993, 0.0013185543793476045, 0.001294420174263172, 0.00127875483607759, 0.0012659041912157889, 0.0012433398248735822, 0.001228894554342046, 0.0012003400138518715, 0.001183988904005212, 0.0011747543964566436, 0.0011585547622780935, 0.0011605046672421217, 0.0011473565792502146, 0.0011370039058606926, 0.0011340652778993677, 0.0011226770617605876, 0.0011216442731143861, 0.0011107600578349525, 0.0011026409620242816, 0.0010866919512238764, 0.0010731362559796018, 0.001051089661012024, 0.0010301832647098524, 0.001009888279286232, 0.0009965887156262153, 0.0009909235256389188, 0.0009767536654130364, 0.0009747817276245561, 0.0009568910741692924, 0.000949947980363763, 0.000956703795161448, 0.0009593917997446279, 0.0009746082191319944, 0.0009815127554947322, 0.0009862085012061277, 0.0009848589907084247, 0.0009587748806599638, 0.0009397330121270677, 0.0009244532483694009, 0.0009160174307072283, 0.0009138141482619988, 0.0009141501488348964, 0.0009184162544694721, 0.0009130457535092251, 0.000912208506180038, 0.0009004897976744733, 0.0008954966088329721, 0.000888658170943591, 0.000878327530378521, 0.0008779392018475493, 0.0008724833236925496, 0.0008753007711193868, 0.0008733894235981503, 0.0008842763929806406, 0.0008803270091975667, 0.0008834474079606231, 0.0008812331091031674, 0.0008784927765619131, 0.0008838109495640858, 0.0008909550928927427, 0.000899184352825675, 0.0009081654828930417, 0.000914194214483801, 0.0009259542345352136, 0.0009387635678511666, 0.0009425339349355657, 0.0009425063939050002, 0.0009326494590656548, 0.0009267529244216092, 0.0009192645182108854, 0.0009126023429171226, 0.0009054058716303917, 0.0008956756255316468, 0.0008975015958581308, 0.0008902445343041561, 0.0008840973762819658, 0.0008824283898297043, 0.0008799772381093866, 0.000884678492026895, 0.0008933897199947213, 0.0008983829088362226, 0.000893860671617389, 0.0008973749071175302, 0.0009013435696219998, 0.0009055848883290665, 0.0009138995254567515, 0.0009202174378684471, 0.000930589389979365, 0.000922150818214136, 0.0009280666315795773, 0.0009267253833910438, 0.0009243623629685353, 0.0009317653919845064, 0.0009418922289233926, 0.0009494384712983037, 0.0009643051195974898, 0.0009718458537662879, 0.0009862966325039368, 0.0009917001827008621, 0.0009979795376697665, 0.001014038712592433, 0.0010172830459930335, 0.0010330585483008768, 0.0010469640146333317, 0.001060098332109956, 0.0010826544361429932, 0.0011030761103072145, 0.0011350760337211167, 0.0011531154087414334, 0.0011576624328877758, 0.0011768364983673857, 0.0011841624124977737, 0.0011999406689086737, 0.0012165093528967996, 0.0012281895039595726, 0.0012561601746017613, 0.0012707651831105765, 0.001307240523991351, 0.001333627585376031, 0.0013666217399933432, 0.0014024911782016796, 0.0014332324765187446, 0.0014678102403935655, 0.0014988241949132272, 0.0015329365153714935, 0.0015343879276822883, 0.0015720971067323913, 0.0016118636007657278, 0.001651087536496926, 0.0016970920739533186, 0.001745473402347502, 0.0017665615694514051, 0.0018051024876245825, 0.0018256783915599696, 0.0018815618966801597, 0.0018972630382054765, 0.0019475088943689358, 0.001967589059754146, 0.0019944801219981727, 0.0020293085092511383, 0.0020797967264835726, 0.002127649267090901, 0.002177592171918141, 0.002209096356781867, 0.0022576126362258207, 0.0022860239633570555, 0.002367479315357191, 0.00239798651491445, 0.002459918030346795, 0.002492961758819125, 0.0025305745442622493, 0.0025619850896220525, 0.0025918974029190997, 0.0026126908809959533, 0.0026649499864937407, 0.002671884817990101, 0.0027487573425041584, 0.0027664331759210126, 0.0028080311484869457, 0.002835572179052315, 0.002897776350687257, 0.0029281981730497637, 0.0029626547563900967, 0.002993387792397992, 0.0030170785868903222, 0.0030149964849795806, 0.0030319039236436605, 0.0030360240618162396, 0.0030334957952103388, 0.0030378693108641195, 0.003026379192912247, 0.0030242502712495446, 0.0030348563221202682, 0.0030418489897808152, 0.0030719182869520852, 0.0030982750532031434, 0.0030908086798168716, 0.0031010319103627363, 0.0031036813575031253, 0.0030762670156783568, 0.003066933360419753, 0.003042223547796504, 0.0030263378813663996, 0.003004663090311454, 0.0029920548065186284, 0.0029706664421815625, 0.0029578268137319874, 0.0029413352446294445, 0.0029132489016588815, 0.0028961762168114094, 0.002857943758180564, 0.00283680050901553, 0.0028030104186148787, 0.0027938640423641197, 0.0027516161014768444, 0.002719478472910115, 0.0026733913123620267, 0.002627637398283779, 0.0025728335015617514, 0.0025436510255746865, 0.002504355483164018, 0.0024615594757684913, 0.002436053727361903, 0.0024182842544411267, 0.0024007185851465346, 0.0023905779776923655, 0.0023550968680150007, 0.002333292634116398, 0.002292746728918062, 0.0022553735504408563, 0.0022384468330553806, 0.002203128215458351, 0.00217902430550754, 0.002143711196116624, 0.0021122262899742946, 0.0020506142504965077, 0.00203825383597877, 0.0020262487007553258, 0.0020074629638066875, 0.0019932738248594093, 0.0019544327094530695, 0.0019488088310116213, 0.0019049882972790627, 0.0018915620448784454, 0.0018528393559035367, 0.001821197465886984, 0.0017890212798774634, 0.0017354539754278208, 0.0016897689139259869, 0.001663423164087155, 0.0016456371665480398, 0.0016412085688331283, 0.001628644350689207, 0.0016130809143167168, 0.0016073331012377244, 0.001603339651805746, 0.0015941712427305346, 0.001588935692820058, 0.0015824029603699523, 0.00157714813173808, 0.0015643332902160138, 0.0015630746651191763, 0.0015527274999357675, 0.0015555421932595482, 0.0015637163711313498, 0.0015732180266764021, 0.001592557338339404, 0.001584653062567143, 0.0015960522951181493, 0.0016165015103129358, 0.0016268707083207973, 0.0016398039762742945, 0.001641899848700319, 0.0016484215647381982, 0.0016487190078683044, 0.0016555629539637985, 0.0016557612493838694, 0.0016741145921526312, 0.0017004658501975761, 0.0017330110860166727, 0.0017605190673453631, 0.0017664348807108045, 0.0017779084740443371, 0.001790398331405732, 0.0018131775177863488, 0.0018366452299310996, 0.0018605453362557267, 0.0018882543671075445, 0.0018984252696953353, 0.001914192509694009, 0.0019416316384462862, 0.0019781785860065308, 0.0020108477564631713, 0.0020298097560074277, 0.0020661143424986973, 0.002068810609391047, 0.002110609631480107, 0.002115869968318093, 0.0021256800834054774, 0.0021556667574850513, 0.002178443189762611, 0.0021840174943490416, 0.002213334921385877, 0.002212183706308245, 0.00223874152208243, 0.0022391546375409104, 0.002258397555596934, 0.0022739802706908193, 0.0023094503639559585, 0.002319709397841558, 0.002351866305129683, 0.002368812301236555, 0.0023749456887434623, 0.002389630566240917, 0.0023986777947816403, 0.00241149814450982, 0.0024190003212358263, 0.0024229882624616918, 0.002422095933071374, 0.002423731870286957, 0.0024201625527256847, 0.0024417767535133868, 0.0024415812121963724, 0.002455808908586442, 0.002457513698378438, 0.0024465385976981386, 0.0024522313287160006, 0.0024169705472831585, 0.0024148361174143426, 0.0023995701241719585, 0.0023793853028705996, 0.0023548297200185167, 0.002332361747283289, 0.0023205108418310103, 0.0022940521737668603, 0.0022523164960481005, 0.0022274744864781374, 0.0022039158889325208, 0.0021684926154193433, 0.0021411526343771015, 0.002118635087786856, 0.002083801192327777, 0.002047124801923875, 0.0020278653592495127, 0.0019697703093749233, 0.0019519264756716211, 0.0019212622922401392, 0.0018812286502103187, 0.0018427428140982722, 0.001812265909674635, 0.00175640994558501, 0.0017214080498394828, 0.0016736711815605288, 0.0016349457384825634, 0.0015946835058990505, 0.0015675610989982752, 0.0015259052902681545, 0.0014996366553149056, 0.001476708747369236, 0.001439175830914751, 0.0014011692087345419, 0.0013630882257718063, 0.0013162216540587178, 0.0012905451512626243, 0.0012539458757443056, 0.0012235736272368167, 0.0012001196856073486, 0.001185272316029558, 0.0011544346241055146, 0.0011379100057662933, 0.0010844501113358553, 0.0010647610285846733, 0.0010130802847287583, 0.0009929670701068693, 0.0009656849252288149, 0.0009476042386626501, 0.0009280005331062204, 0.0009123489654359212, 0.0008921173243826012, 0.0008740696870531149, 0.000861342976828858, 0.0008399518583887359, 0.0008269304591374295, 0.000805963472568014, 0.0007840931401960546, 0.0007730684656607372, 0.0007618757908389714, 0.000755502796366145, 0.0007484440302322409, 0.0007361304354664644, 0.0007236515945172958, 0.0007035631668229157, 0.0006909796699575985, 0.0006775396470416985, 0.0006603843391025302, 0.0006506954045496334, 0.0006404831904159946, 0.0006315406177914192, 0.000626814576946402, 0.0006201799426832045, 0.0006156053775062967, 0.0006078663479174281, 0.0005998298751984535, 0.0005900335306263518, 0.0005812644664943382, 0.0005748804556092857, 0.0005698349388097101, 0.000566761359798615, 0.0005616442363195694, 0.0005622749259195163, 0.0005532993040582626, 0.0005422911541412846, 0.0005348495676825219, 0.0005325361211150309, 0.0005320376284617976, 0.0005307018884793774, 0.0005264054877111798, 0.0005264054877111798, 0.0005228637111804734, 0.0005181238998201733, 0.0005176309153730532, 0.0005136154331166225, 0.0005124091359778592, 0.0005101562796776121, 0.0005055431570579128, 0.0004995529829099451, 0.0004920150028442035, 0.0004884759804165536, 0.00048560345092858563, 0.000481450263519328, 0.000479029406932632, 0.00047415189041950524, 0.00047243608421528277, 0.0004715299843096821, 0.00047353772543789753, 0.00047000971942247376, 0.0004698554896513077, 0.0004721276246729506, 0.0004682388311571205, 0.0004696351614067847, 0.0004644106279085342, 0.00046173088563452376, 0.0004594807834373332, 0.0004550053659704607, 0.0004509155229315034, 0.00044808430498938354, 0.0004430277717775818, 0.0004410696045043841, 0.00043787759906185783, 0.00043347929648056836, 0.0004299017166101269, 0.00042542354504019795, 0.00042215993291820175, 0.00041868425486085215, 0.000416883071461877, 0.0004110388647759057, 0.0004118981449295452, 0.00040788541677617095, 0.00040867033614728403, 0.00040761000647051725, 0.0004041866563712419, 0.00040178507850594175, 0.00039903372955246133, 0.0003977007436730975, 0.0003977310388067194, 0.00039884645054461687, 0.00039690480788975835, 0.000394671230310907, 0.0003933712936682215, 0.00039117076532604856, 0.0003899947633209073, 0.00038895095826247983, 0.00038990112381698505, 0.00038822662915861066, 0.0003852577060636639, 0.00038354740806555447, 0.0003831673418437523, 0.00038108523993301045, 0.00038199133983861106, 0.0003807712721845652, 0.0003789921216100424, 0.0003772350038599718, 0.00037759028315426514, 0.0003756155912627282, 0.0003736216206497954, 0.000373136898511845, 0.0003710079768491419, 0.0003707132878220925, 0.0003699917128212798, 0.00036924259678990177, 0.0003697686304737003, 0.000369484957858877, 0.0003692976788510325, 0.00037006056539769325, 0.00036974108944313496, 0.00036845492331573224, 0.0003671825277036122, 0.0003674441674939832, 0.00036729820003198675, 0.00036671708428705744, 0.0003670723635813507, 0.0003662516408705027, 0.0003653593114801848, 0.0003654336722627113, 0.00036621859163382426, 0.0003649076385789127, 0.0003645000313265452, 0.00036404009611610357, 0.00036481399907499045, 0.00036354435756592694, 0.0003624454704463687, 0.00036318632416857717, 0.000362616224835874, 0.00036201858447260554, 0.0003629026515537539, 0.00036316429134412485, 0.0003618092726403087, 0.00036178173160974337, 0.0003609059268377646, 0.0003606580575626763, 0.00035972441662651027, 0.00035978776099681063, 0.0003598290725426587, 0.0003593278257863689, 0.00035902487445014993, 0.0003587962838964574, 0.00035836939792269413, 0.00035583837721373673, 0.0003554059830338604, 0.0003547532606094612, 0.0003549102444836838, 0.00035429057129596295, 0.0003543126041204152, 0.0003549185067928534, 0.0003548248672889311, 0.00035513057272820676, 0.0003544998831282598, 0.00035434014515098067, 0.000354516407746599, 0.00035333489753534467, 0.0003535855209134895, 0.0003530154215807864, 0.0003527152243476239, 0.0003532798154742139, 0.00035263260125592777, 0.0003519964034498677, 0.000351608074918896, 0.00035093882787615757, 0.000349443349916458, 0.00034942957940117537, 0.0003491624314046913, 0.00034956453045094566, 0.00034901095573658175, 0.00034910184113744744, 0.0003489310867479422, 0.0003488181685226241, 0.0003479836752964935, 0.0003476917403725006, 0.00034843259409470895, 0.0003489586277785075, 0.0003480910853156984, 0.0003474548875096384, 0.0003469619030625183, 0.00034665344352018617, 0.0003463918037298151, 0.00034654052529486815, 0.00034605304905386115, 0.0003454196053508576, 0.00034516347376659963, 0.00034559862204953256, 0.0003448357355028718, 0.0003449403914190202, 0.00034430419361296017, 0.00034424635744877293, 0.000344852260121211, 0.0003448384896059283, 0.0003451028834993559, 0.0003437423565894266, 0.0003425580922751158, 0.00034259664971790727, 0.0003416354677511759, 0.00034174838597649394, 0.00034173461546121124, 0.0003417869434192854, 0.0003409965158420593, 0.00034094143378092864, 0.0003408477942770064, 0.0003402501539137379, 0.0003404980231888262, 0.0003398783500011054, 0.00033904936498108774, 0.00033842969179336696, 0.00033828372433137053, 0.0003380661501899041, 0.00033740791955939176, 0.000338358085113897, 0.0003377081167925543, 0.00033727847671573453, 0.000337388640837996, 0.00033701959102842003, 0.00033749605085720095, 0.00033774116602923275, 0.0003364384752834908, 0.000335931720321088, 0.0003357031297673954, 0.00033592070390886183, 0.0003353395881639325, 0.00033492922680850853, 0.00033513303043469225, 0.00033468961984258985, 0.0003348713906443213, 0.00033494024322073466, 0.0003348108003770775, 0.00033487689885043436, 0.00033441145543387964, 0.0003341993894985263, 0.0003345464064836499, 0.00033424896335354395, 0.00033390194636842026, 0.00033334837165405635, 0.00033337040447850867, 0.0003331583385431553, 0.0003329132233711235, 0.0003332326993256818, 0.0003335301424557878, 0.0003335026014252224, 0.00033401761869679484, 0.0003333428634479433, 0.00033282509207331433, 0.00033313630571870306, 0.0003330839777606288, 0.00033270666564188324, 0.00033214758272140626, 0.00033204843501137094, 0.00033124974512497527, 0.0003311781384455053, 0.00033189695934326144, 0.0003313213518044452, 0.0003320980088663886, 0.0003318336149729611, 0.00033207873014499283, 0.0003325304030462649, 0.0003314094831022544, 0.00033175650008737803]]
  out "Camera Status:":bool
  out "Raw Image":i32[][](graph)
  out "VBI":i32[](graph)
  out "Bits/pixel":u16
  out "BufNr1":i16
  out "BufNr0":i16
  in  "ExposureTimeBase":u16(ring)=2 items=["nanoseconds", "microseconds", "milliseconds"]
  in  "Xmin":u16=760 min=1
  in  "Ymin":u16=410 min=1
  in  "Ymax":u16=1200 min=1
  in  "Xmax":u16=1560 min=1
  in  "Rate":i32(ring) items=["204000000", "0", "0", "0"]
  out "YResAct":u16
  out "XResAct":u16
  in  "Buffer0":bool
  in  "Buffer1":bool
  out "Horizontal resolution":u16
  out "Vertical resolution":u16
  in  "Exposure Time (secs)":sgl format="%.2f"
  out "Detector X Pixels":i32
  out "Detector Y Pixels":i32
  in  "Trigger":u32(ring) items=["Internal", "External"]
  out "Camera inputs":T6
  out "Camera outputs":T7
  out "Start Acquisition":u32
  out "Get Status":u32
  out "Status":u32
  out "Get Acquired Data":u32
  out "Shut Down":u32
  out "Image buffer":u64[](array[numeric])
  out "End of scan":bool
  # "Image Settings"
  # "Pump - probe scan Settings"
  # "Program Control"
  # "Analysis Settings"
  # "Saving Settings"
  # "Scan parameters"
  # "Y axis"
  # "VMI camera"
  # "XUV camera"
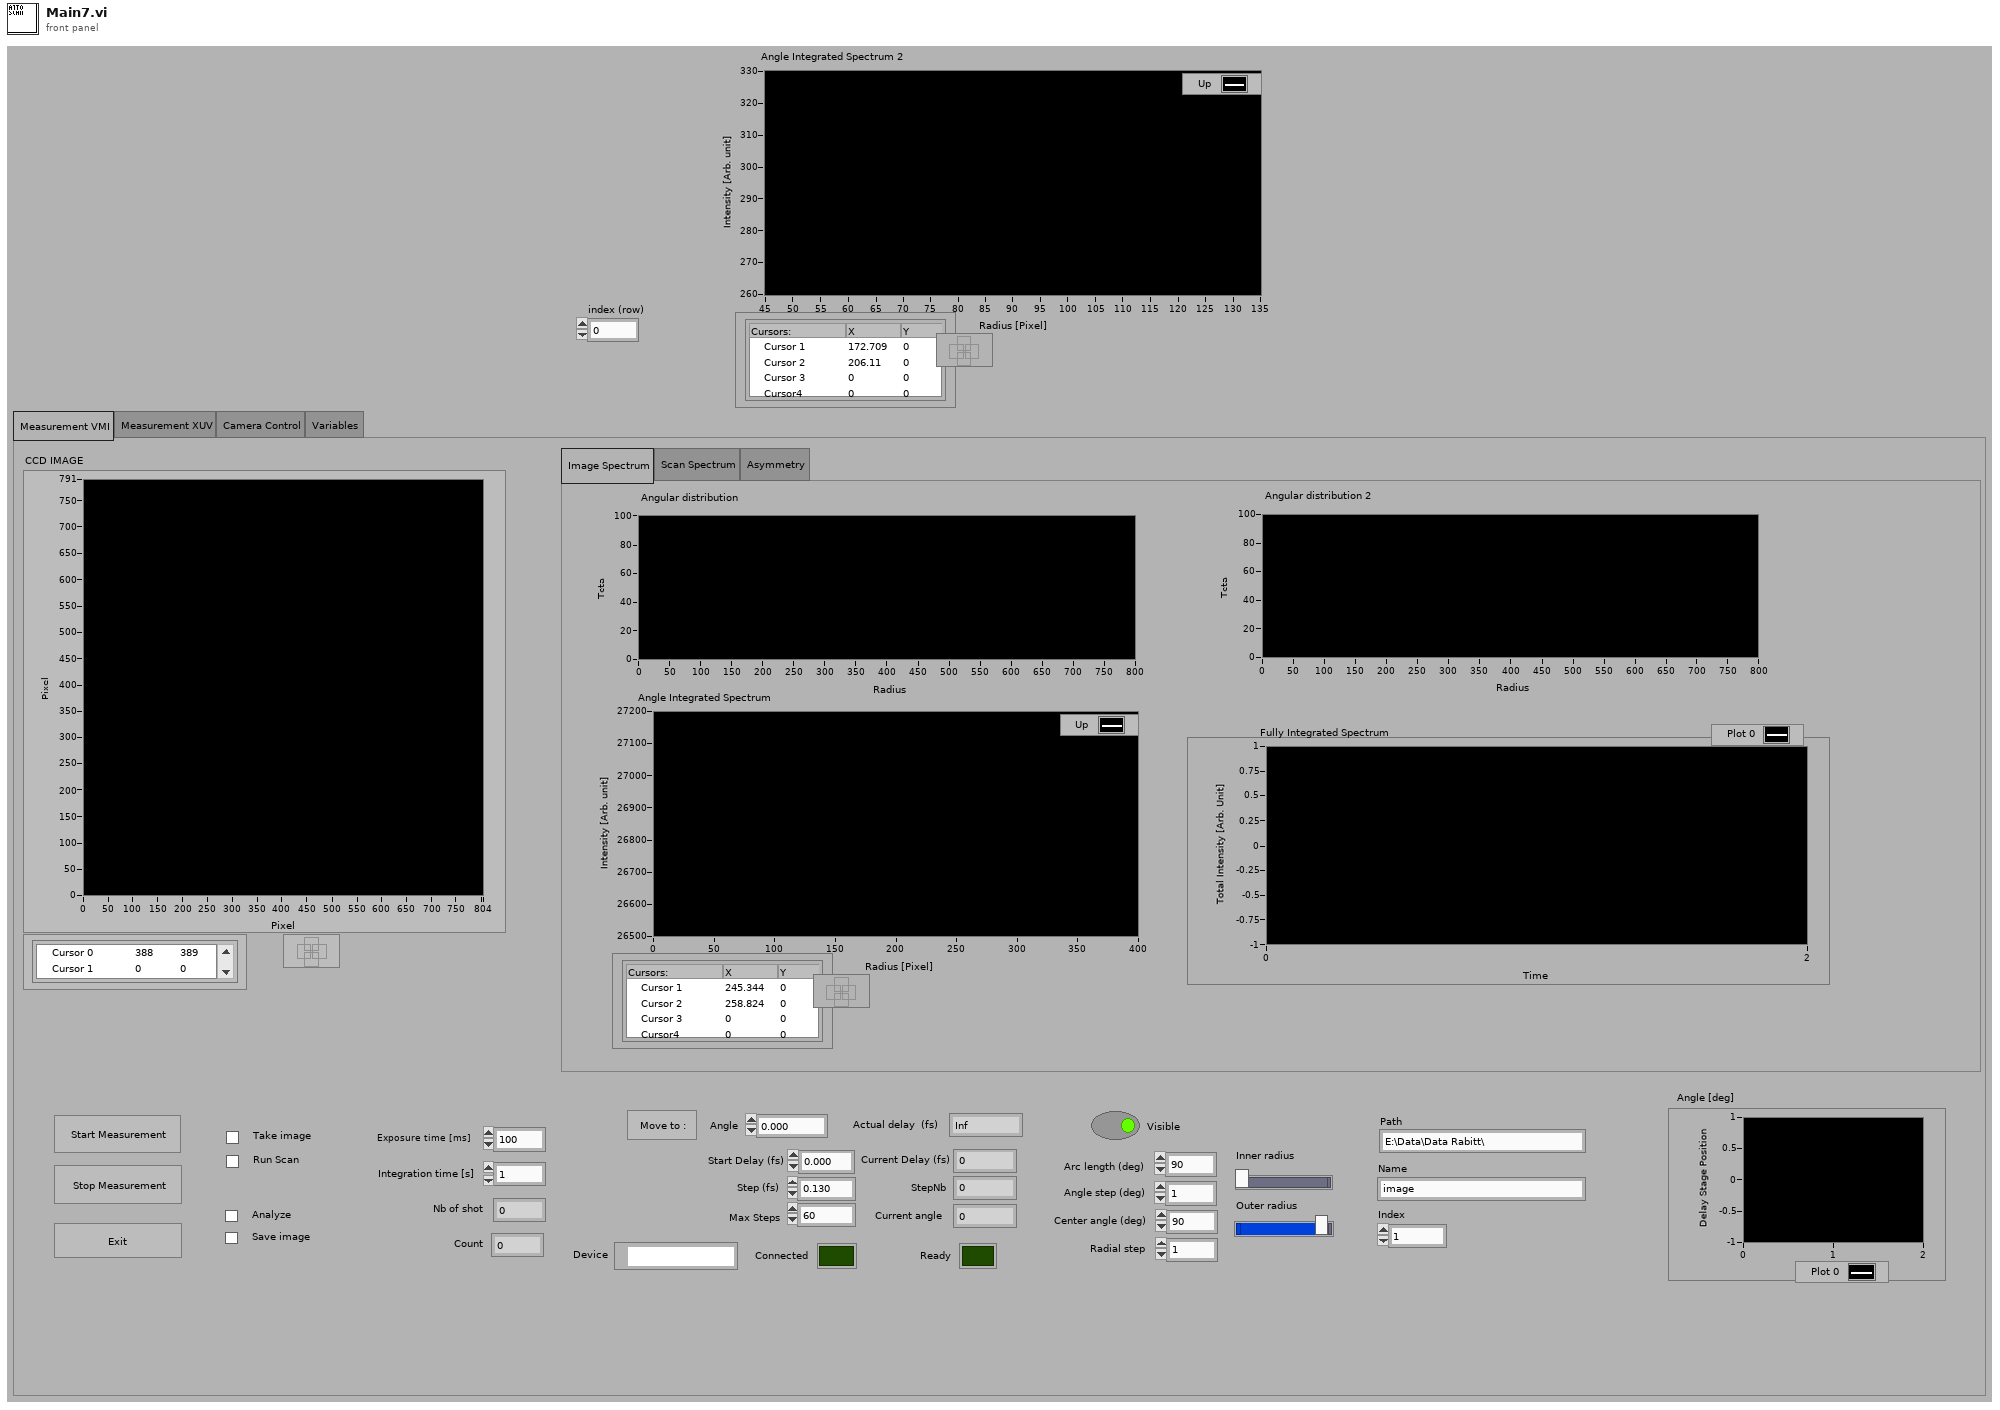
[diagram p1: front panel]
types:
  T1 = cluster{"Angle Sampling":dbl[], "Angle versus Radius Distribution":dbl[]}
  T2 = cluster{"Center angle (deg)":dbl, "Arc length (deg)":dbl, "Angle step (deg)":dbl, "Outer radius ":dbl, "Inner radius ":dbl, "Radius":dbl, "Radial step ":dbl}
  T3 = enum32{"Measurement VMI", "Measurement XUV", "Camera Control", "Variables"}
  T4 = enum32{"Image Spectrum", "Scan Spectrum", "Asymmetry"}
  T5 = cluster{"Radius Sampling":dbl[], "Angle Integrated Distribution":dbl[]}[]
  T6 = cluster{"Calculated Exposure Value":sgl, "Detector X Pixels":i32, "Detector Y Pixels":i32}
  T7 = cluster{"Initialize":u32, "Set Acquisition Mode":u32, "Set Readout Mode":u32, "Set Gate Mode":u32, "Get Detector":u32, "Set Image":u32, "Set Trigger Mode":u32, "Set Exposure Time":u32, "Check Timings":u32}
  T8 = cluster{"VISA resource name":refnum<visa-resource-name>, "Device name":string, "Controller address":i32, "error":errorcluster}
  T9 = typedef "LVRectTypeDef.ctl" = cluster{"Left":i16, "Top":i16, "Right":i16, "Bottom":i16}
  T10 = cluster{"to shutdown":bool, "to get acquired data":bool, "to start acquisition":bool, "DRV_SUCCESS":i32}
  T11 = cluster{"Size":u16, "SensorTypeDESC":u16, "SensorSubtypeDESC":u16, "MaxHorizontalResStdDESC":u16, "MaxVerticalResStdDESC":u16, "MaxHorizontalResExtDESC":u16, "MaxVerticalResExtDESC":u16, "DynResDESC":u16, "MaxBinHorzDESC":u16, "BinHorzStepDESC":bool, "MaxBinVertDESC":u16, "BinVertStepDESC":bool, "ROIHorzStepDESC":u16, "ROIVertStepDESC":u16, "NumADCDESC":u16, "IRDESC":bool, "MinDelayDESC":u32, "MaxDelayDESC":u32, "MinDelayStepDESC":u32, "MinExpoDESC":u32, "MaxExpoDESC":u32, "MinExpoStepDESC":u32, "MinDelayIRDESC":u32, "MaxDelayIRDESC":u32, "MinExpoIRDESC":u32, "MaxExpoIRDESC":u32, "TimeTableDESC":bool, "DoubleImageDESC":bool, "MinCoolSetDESC":i16, "MaxCoolSetDESC":i16, "MDefaultCoolSetDESC":i16, "PowerDownModeDESC":bool, "OffsetRegDESC":bool, "ColorPattern":cluster{"UpperLeftColor":u8, "UpperRightColor":u8, "LowerLeftColor":u8, "LowerRightColor":u8}, "PatternTypeDESC":bool, "PixelRates":u32[], "CoversionFactors":u16[], "Reserved":u32[], "GeneralCapabilities":u32, "GeneralCapabilities 2":u32, "Min Size Hor":u16, "Min Size Vert":u16, "Ext Synch Freq":u32[], "Cooling Setpoints":i16[], "Soft ROI Hor Step":u16, "Soft ROI Vert Step":u16}
  T12 = typedef "LVCursorListTypeDef.ctl" = cluster{"Name":string, "Color":u32, "Style":u8, "Point Style":u8, "Name Visible":bool, "Allow Drag":bool, "Cursor Mode":u32, "Plot":i32, "Index":i32, "Position":cluster{"X":dbl, "Y":dbl}, "X Scale":u32, "Y Scale":u32, "Watch Plots":i32[], "Watch All Plots":bool, "Plot Area":i32, "Label Offset":cluster{"X":dbl, "Y":dbl}}[]
  T13 = cluster{"Name":string, "Color":u32, "Style":u8, "Point Style":u8, "Name Visible":bool, "Allow Drag":bool, "Cursor Mode":u32, "Plot":i32, "Index":i32, "Position":cluster{"X":dbl, "Y":dbl}, "X Scale":u32, "Y Scale":u32, "Watch Plots":i32[], "Watch All Plots":bool, "Plot Area":i32, "Label Offset":cluster{"X":dbl, "Y":dbl}}
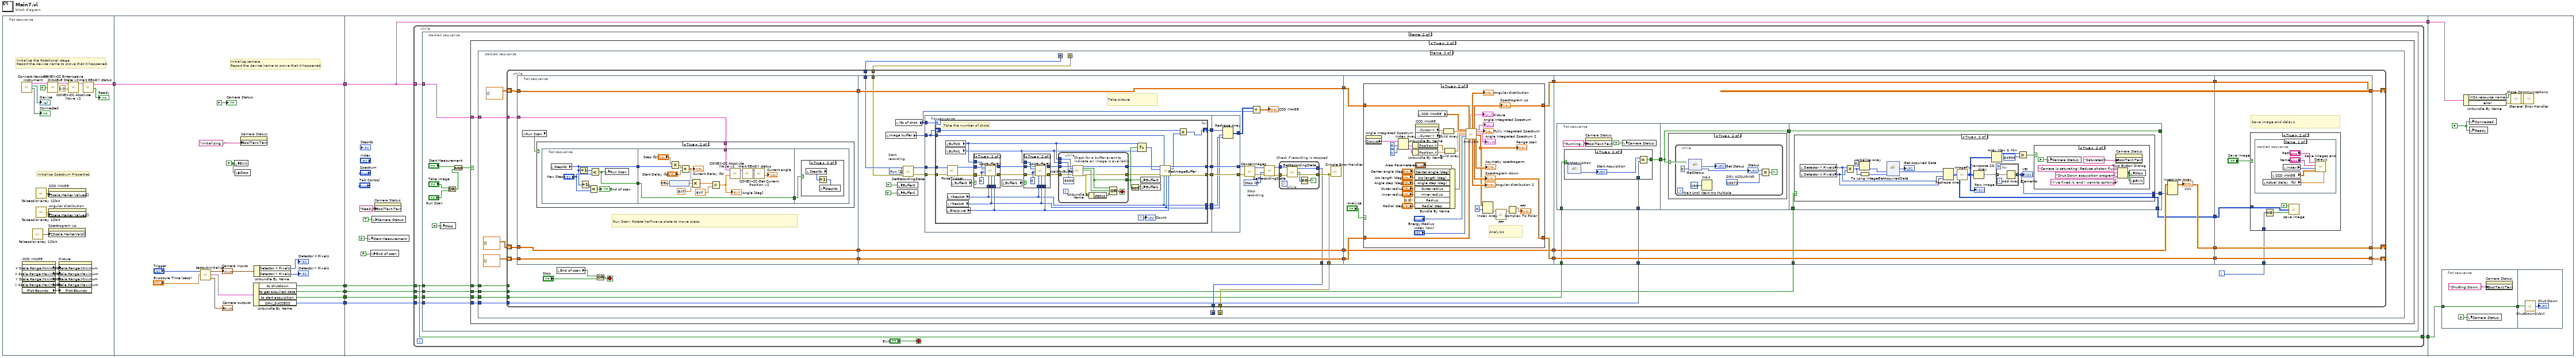
[diagram p0: block diagram]
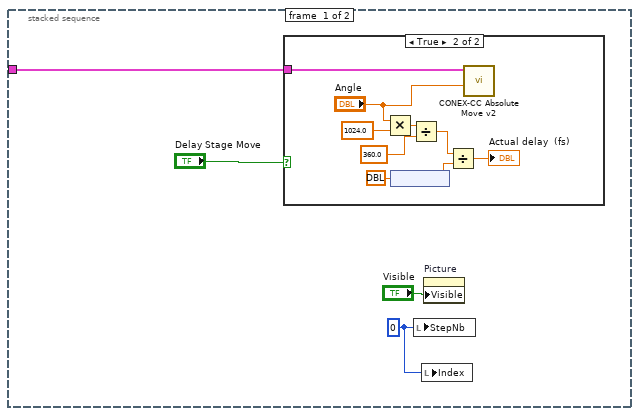
[diagram p2: hidden frame]
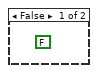
[diagram p4: hidden frame]
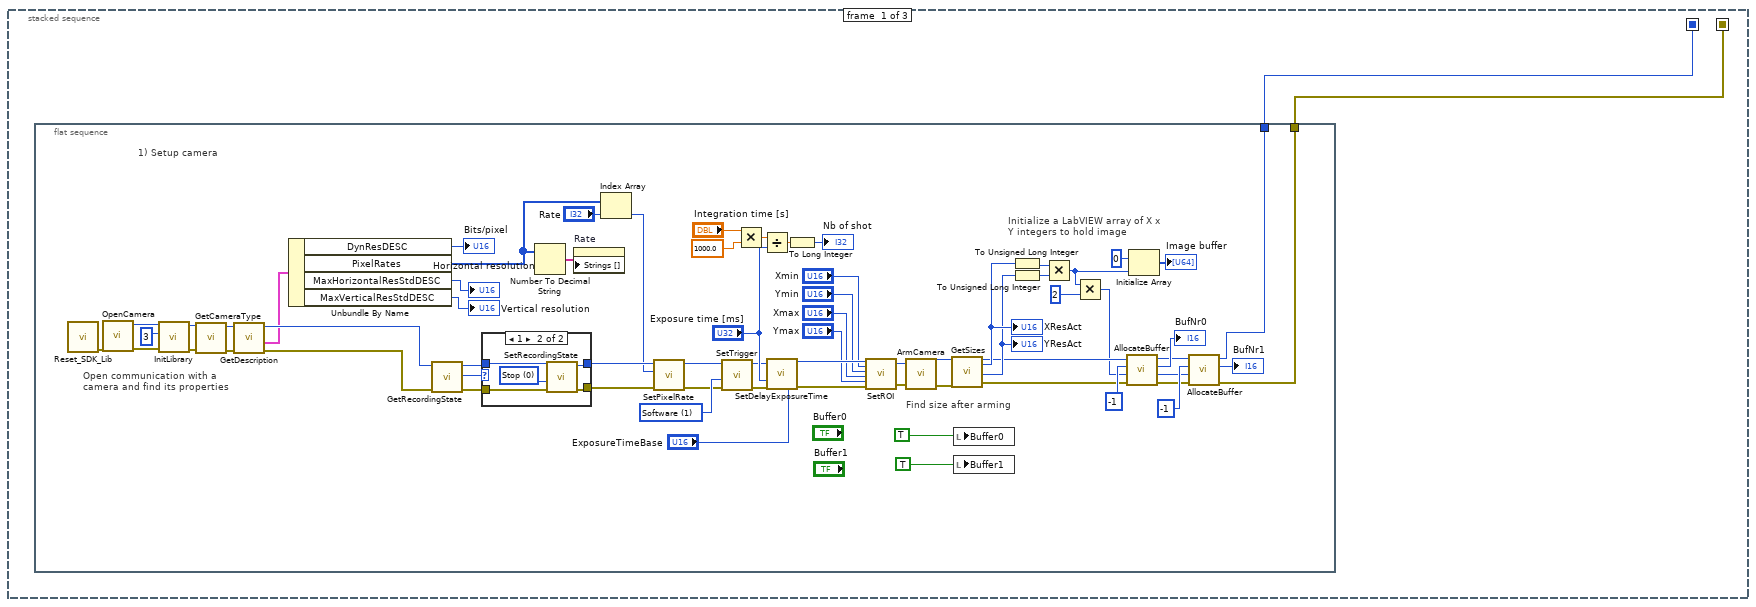
[diagram p5: hidden frame]
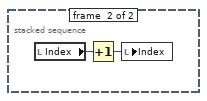
[diagram p17: hidden frame]
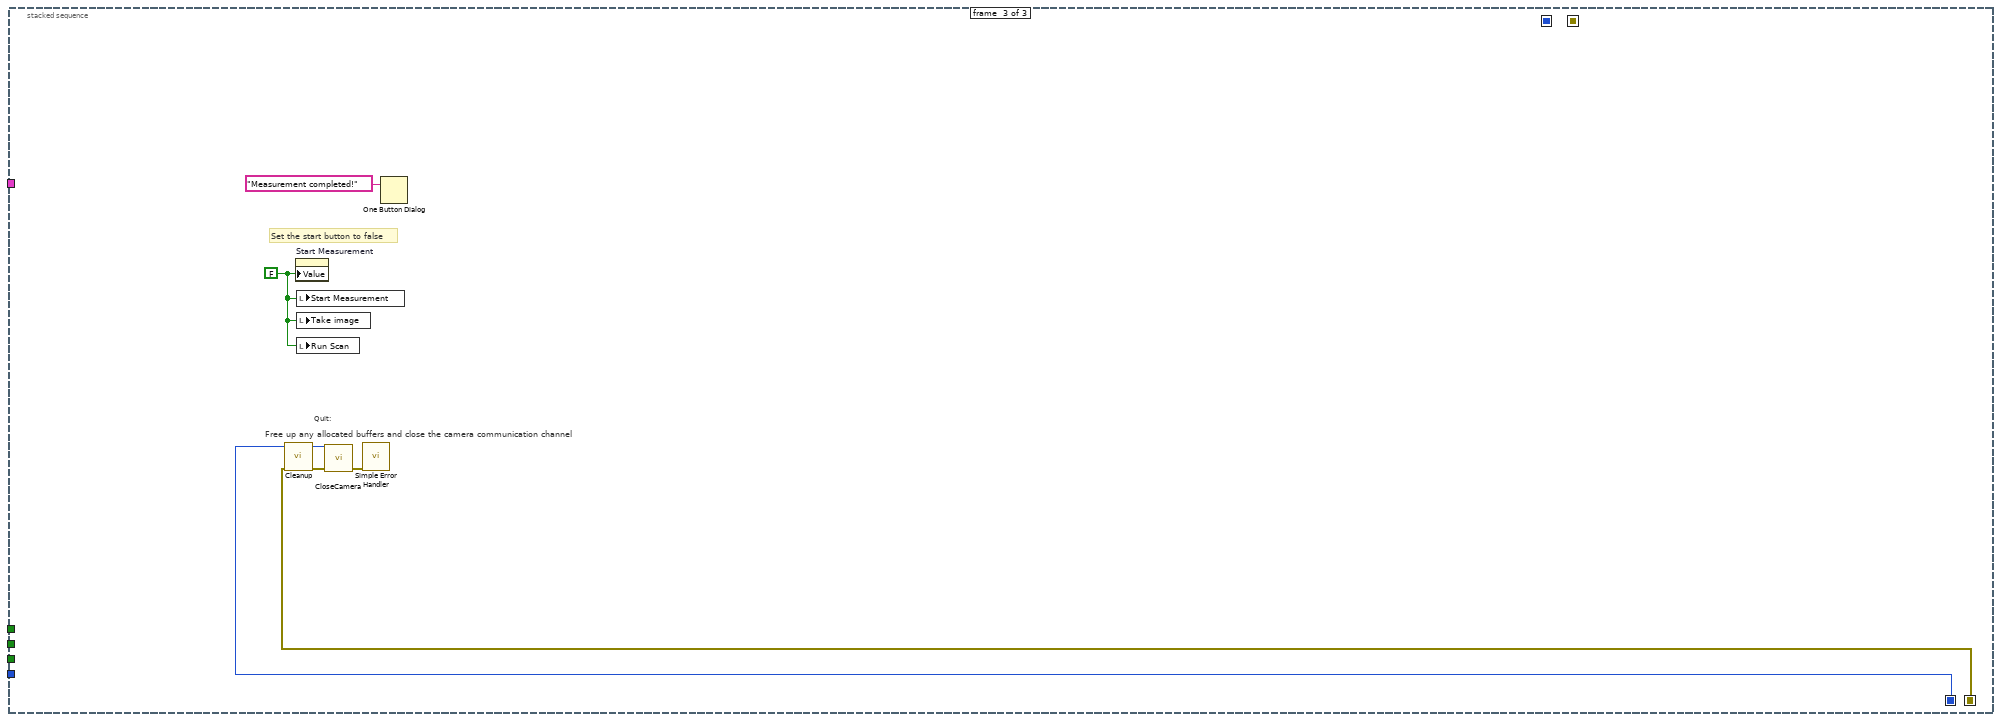
[diagram p18: hidden frame]
diagram:
  n1 = flat-sequence {
    tunnel: [w11] -> w7
    tunnel: w7 -> [w40]
    tunnel: [w40] -> w6
    tunnel: [w30] -> w5
    tunnel: [w29] -> w4
    tunnel: [w28] -> w3
    tunnel: [w27] -> w2
    tunnel: w6 -> [w49]
    tunnel: [w49] -> w8
    tunnel: w5 -> [w48]
    tunnel: w4 -> [w47]
    tunnel: w3 -> [w46]
    tunnel: w2 -> [w45]
    tunnel: [w44] -> w1
    tunnel: w8 -> [w475]
    tunnel: w1 -> [w472]
    frame #0 {
      # "Initialize Spectrum Properties"
      # "Initialize the Rotational stage.\nReport the device name to prove that it happened."
      n2 = call <userlib>:"Connect Newport Instrument.vi"() -> ("Connected"=→"Connected":bool, "VISA resource name (duplicate)"=→"Device":refnum<visa-resource-name>, "Device Connection Cluster"=w15:T8)  [unwired: 7 in, 2 out]
      n3 = property on="CCD IMAGE" class="IntGraph (strict)"() -> ("X Scale.Range:Minimum"=w21:dbl, "X Scale.Range:Maximum"=w20:dbl, "Y Scale.Range:Minimum"=w19:dbl, "Y Scale.Range:Maximum"=w18:dbl, "Plot Bounds"=w22:T9)  [unwired: 2 in, 2 out]
      n4 = call "falsecolor array 12bit.vi"() -> ("Color Array"=w23:cluster{dbl, u32}[])  [unwired: 1 in]
      n5 = call "falsecolor array 12bit.vi"() -> ("Color Array"=w25:cluster{dbl, u32}[])  [unwired: 1 in]
      n6 = call "falsecolor array 12bit.vi"() -> ("Color Array"=w24:cluster{dbl, u32}[])  [unwired: 1 in]
      n7 = call <userlib>:"CONEX-CC Enter-Leave DISABLE State v2.vi"("Ready? (false=DISABLE true=READY)"=TRUE, "Connection Cluster in"=w15) -> ("Connection Cluster out"=w14:T8)  [unwired: 7 in]
      n8 = property on="Spectrogram up" class="IntGraph (strict)"("ZScale.MarkerVals[]"=w23) -> ()  [unwired: 2 in, 2 out]
      n9 = property on="CCD IMAGE" class="IntGraph (strict)"("Z Scale.Marker Values[]"=w25) -> ()  [unwired: 2 in, 2 out]
      n10 = property on="Angular distribution" class="IntGraph (strict)"("Z Scale.Marker Values[]"=w24) -> ()  [unwired: 2 in, 2 out]
      n11 = property on="Picture" class="XYGraph (strict)"("X Scale.Range:Minimum"=w21, "X Scale.Range:Maximum"=w20, "Y Scale.Range:Minimum"=w19, "Y Scale.Range:Maximum"=w18, "Plot Bounds"=w22) -> ()  [unwired: 2 in, 2 out]
      n12 = call <userlib>:"CONEX-CC Absolute Move v2.vi"("Target position"=0.0, "Connection Cluster in"=w14) -> ("Connection Cluster out"=w13:T8)  [unwired: 7 in]
      n13 = call <userlib>:"Wait READY status.vi"("Connection Cluster in"=w13) -> ("IsReady?"=→"Ready":bool, "Connection Cluster out"=w11:T8)  [unwired: 9 in]
    }
    frame #1 {
      w26 = FALSE ("Exit")
      # "Initialize camera\nReport the device name to prove that it happened."
      n14 = call "testsubinitialize.vi"("Exposure Time (secs)"="Exposure Time (secs)", "Trigger"="Trigger") -> ("Camera outputs"=→"Camera outputs":T7, "Camera status"=w33:T10, "Camera inputs"=w36:T6)  [unwired: 1 in]
      "Camera inputs" <- w36
      n15 = local write "Exit"(w26) -> ()
      n16 = local write "Stop"(w26) -> ()
      n17 = property on="Camera Status:" class="Bool (strict)"("BoolText.Text"="Initializing..." ("String")) -> ()  [unwired: 2 in, 2 out]
      n18 = Unbundle By Name(w33) -> ("to shutdown"=w30:bool, "to get acquired data"=w29:bool, "to start acquisition"=w28:bool, "DRV_SUCCESS"=w27:i32)
      n19 = Unbundle By Name(w36) -> ("Detector X Pixels"=→"Detector X Pixels":i32, "Detector Y Pixels"=→"Detector Y Pixels":i32)
      "Camera Status:" <- FALSE ("Camera Status:")
    }
    frame #2 {
      n20 = local write "Start Measurement"(FALSE) -> ()
      n21 = local write "End of scan"(FALSE) -> ()
      n22 = local write "Camera Status:"(TRUE ("Camera Status:")) -> ()
      n23 = property on="Camera Status:" class="Bool (strict)"("BoolText.Text"="Ready" ("Boolean Text.Text")) -> ()  [unwired: 2 in, 2 out]
      n24 = while {
        tunnel: w49 -> [w55]
        tunnel: w48 -> [w51]
        tunnel: w47 -> [w54]
        tunnel: w46 -> [w53]
        tunnel: w45 -> [w52]
        tunnel: [w51] -> w44
        stop <- "Exit" stop-if-true
        n25 = stacked-sequence {
          tunnel: w55 -> [w58 w75]
          tunnel: w51 -> [_ w74]
          tunnel: w54 -> [_ w73]
          tunnel: w53 -> [_ w72]
          tunnel: w52 -> [_ w71]
          frame #0 {
            w57 = 0 ("Done Step")
            n26 = case shown="True" "Delay Stage Move" {
              tunnel: w58 -> [_ w63]
              frame False {
              }
              frame True {
                n27 = Multiply(x="Angle", y=1024.0) -> (x*y=w68:dbl)
                n28 = node(ext[unit] 299792458.0) -> (w64:ext)
                n29 = Divide(x=w68, y=360.0) -> (x/y=w66:dbl)
                n30 = Divide(x=w66, y=w64) -> (x/y=→"Actual delay  (fs)":ext)
                n31 = call <userlib>:"CONEX-CC Absolute Move v2.vi"("Target position"="Angle", "Connection Cluster in"=w63) -> ()  [unwired: 7 in, 1 out]
              }
            }
            n32 = local write "StepNb"(w57) -> ()
            n33 = local write "Index"(w57) -> ()
            n34 = property on="Picture" class="XYGraph (strict)"("Visible"="Visible") -> ()  [unwired: 2 in, 2 out]
          }
          frame #1 {
            n35 = local write "Stop"(FALSE ("Stop")) -> ()
            n36 = Or(x="Take image", y="Run Scan") -> (x .or. y?=w76:bool)
            n37 = And(x="Start Measurement", y=w76) -> (x .and. y?=w78:bool)
            n38 = case shown="True" w78 {
              tunnel: w75 -> [_ w85]
              tunnel: w74 -> [_ w84]
              tunnel: w73 -> [_ w83]
              tunnel: w72 -> [_ w82]
              tunnel: w71 -> [_ w81]
              frame False {
                (unwired) FALSE
              }
              frame True {
                n39 = stacked-sequence {
                  seq-local: [_ w170 _] -> [_ _ w467]
                  seq-local: [_ w169 _] -> [_ _ w466]
                  seq-local: [w86 _ _] -> [_ w167 _]
                  seq-local: [w87 _ _] -> [_ w168 _]
                  tunnel: w85 -> [_ w166 _]
                  tunnel: w84 -> [_ w165 _]
                  tunnel: w83 -> [_ w164 _]
                  tunnel: w82 -> [_ w163 _]
                  tunnel: w81 -> [_ w162 _]
                  frame #0 {
                    n40 = flat-sequence {
                      tunnel: [w89] -> w86
                      tunnel: [w88] -> w87
                      frame #0 {
                        w125 = u16 1 items=["Auto", "Software", "External sequence start ", "External exposure control"] ("TriggerMode")
                        # "Find size after arming"
                        # "1) Setup camera"
                        # "Initialize a LabVIEW array of X x Y integers to hold image"
                        # "Open communication with a camera and find its properties"
                        n41 = call "Reset_SDK_Lib.vi"() -> ("ErrorOut"=w110:errorcluster)  [unwired: 11 in]
                        n42 = call "OpenCamera.vi"("ErrorIn"=w110) -> ("ErrorOut"=w101:errorcluster, "Handle out"=w100:u64)  [unwired: 3 in, 2 out]
                        n43 = call "InitLibrary.vi"("error in (no error)"=w101, "InterfaceType"=u32 3, "ph"=w100) -> ("error out"=w102:errorcluster, "hout"=w103:u64)  [unwired: 7 in]
                        n44 = call "GetCameraType.vi"("ph"=w103, "error in (no error)"=w102) -> ("hout"=w94:u64, "error out"=w95:errorcluster)  [unwired: 1 in, 2 out]
                        n45 = call "GetDescription.vi"("ErrorIn"=w95, "ph"=w94) -> ("ErrorOut"=w105:errorcluster, "Description"=w93:T11, "hout"=w106:u64)  [unwired: 2 in, 1 out]
                        n46 = Unbundle By Name(w93) -> ("DynResDESC"=→"Bits/pixel":u16, "PixelRates"=w124:u32[], "MaxHorizontalResStdDESC"=→"Horizontal resolution":u16, "MaxVerticalResStdDESC"=→"Vertical resolution":u16)
                        n47 = call "GetRecordingState.vi"("ErrorIn"=w105, "ph"=w106) -> ("ErrorOut"=w108:errorcluster, "Error"=w109:i32, "hout"=w107:u64)  [unwired: 2 in, 1 out]
                        n48 = case shown="1" w109 {
                          tunnel: w107 -> [w155 w159]
                          tunnel: w108 -> [w154 w158]
                          tunnel: [w155 w157] -> w142
                          tunnel: [w154 w156] -> w143
                          frame 0, Default {
                          }
                          frame 1 {
                            w160 = u16 0 items=["Stop", "Run"] ("RecordingState")
                            n49 = call "SetRecordingState.vi"("ErrorIn"=w158, "RecordingState"=w160, "ph"=w159) -> ("ErrorOut"=w156:errorcluster, "hout"=w157:u64)  [unwired: 2 in, 1 out]
                          }
                        }
                        n50 = Number To Decimal String(number=w124) -> (decimal integer string=w99:string[])  [unwired: 1 in]
                        n51 = property on="Rate" class="Ring (strict)"("Strings []"=w99) -> ()  [unwired: 2 in, 2 out]
                        n52 = Index Array(array=w124, index="Rate") -> (element=w123:u32)
                        n53 = call "SetPixelRate.vi"("error in (no error)"=w143, "PixelRate"=w123, "ph"=w142) -> ("error out"=w114:errorcluster, "hout"=w115:u64)  [unwired: 2 in, 1 out]
                        n54 = call "SetTrigger.vi"("error in (no error)"=w114, "TriggerMode"=w125, "ph"=w115) -> ("error out"=w121:errorcluster, "hout"=w122:u64)  [unwired: 2 in, 1 out]
                        n55 = Multiply(x="Integration time [s]", y=1000.0) -> (x*y=w149:dbl)
                        n56 = Divide(x=w149, y="Exposure time [ms]") -> (x/y=w151:dbl)
                        n57 = call "SetDelayExposureTime.vi"("ph"=w122, "Exposure"="Exposure time [ms]", "error in (no error)"=w121, "ExposureTimeBase"="ExposureTimeBase") -> ("hout"=w119:u64, "error out"=w118:errorcluster)  [unwired: 9 in, 1 out]
                        n58 = To Long Integer(number=w151) -> (32bit integer=→"Nb of shot":i32)
                        n59 = call "SetROI.vi"("ph"=w119, "ROIX0"="Xmin", "ROIY0"="Ymin", "ROIX1"="Xmax", "ROIY1"="Ymax", "error in (no error)"=w118) -> ("hout"=w136:u64, "error out"=w137:errorcluster)  [unwired: 12 in]
                        n60 = call "ArmCamera.vi"("error in (no error)"=w137, "ph"=w136) -> ("error out"=w134:errorcluster, "hout"=w135:u64)  [unwired: 1 in, 1 out]
                        n61 = call "GetSizes.vi"("ph"=w135, "ErrorIn"=w134) -> ("hout"=w132:u64, "XResAct"=w153:u16, "YResAct"=w152:u16, "ErrorOut"=w133:errorcluster)  [unwired: 11 in, 3 out]
                        "YResAct" <- w152
                        "XResAct" <- w153
                        n62 = local write "Buffer0"(TRUE) -> ()
                        n63 = local write "Buffer1"(TRUE) -> ()
                        n64 = To Unsigned Long Integer(number=w153) -> (unsigned 32bit integer=w129:u32)
                        n65 = To Unsigned Long Integer(number=w152) -> (unsigned 32bit integer=w130:u32)
                        n66 = Multiply(x=w129, y=w130) -> (x*y=w139:u32)
                        n67 = Multiply(x=w139, y=u32 2) -> (x*y=w126:u32)
                        n68 = call "AllocateBuffer.vi"("error in (no error)"=w133, "Size"=w126, "BufNr"=i16 -1, "ph"=w132) -> ("error out"=w128:errorcluster, "BufNrOut"=→"BufNr0":i16, "hout"=w127:u64)  [unwired: 2 in, 3 out]
                        n69 = Initialize Array(u16 0 ("Element Data"), w139) -> (→"Image buffer":u16[])
                        n70 = call "AllocateBuffer.vi"("error in (no error)"=w128, "Size"=w126, "BufNr"=i16 -1, "ph"=w127) -> ("error out"=w88:errorcluster, "BufNrOut"=→"BufNr1":i16, "hout"=w89:u64)  [unwired: 2 in, 3 out]
                      }
                    }
                  }
                  frame #1 {
                    n71 = while {
                      shift-right: [w202] -> _
                      shift-left: dbl[][] [] -> [w203]
                      shift-right: [w200] -> _
                      shift-left: dbl[][] [] -> [w201]
                      tunnel: [w192] -> w170
                      tunnel: [w191] -> w169
                      tunnel: w167 -> [w190]
                      tunnel: w168 -> [w189]
                      tunnel: w166 -> [w188]
                      tunnel: w165 -> [_]
                      tunnel: w164 -> [w181]
                      tunnel: w163 -> [w182]
                      tunnel: w162 -> [w183]
                      shift-right: [w175] -> _
                      shift-left: dbl[][] [] -> [w180]
                      i -> [w173]
                      stop <- w199 stop-if-true
                      n72 = flat-sequence {
                        tunnel: w203 -> [w207]
                        tunnel: [w207] -> w196
                        tunnel: w201 -> [w206]
                        tunnel: [w206] -> w195
                        tunnel: w188 -> [w205]
                        tunnel: w180 -> [w204]
                        tunnel: [w204] -> w177
                        tunnel: w196 -> [w248]
                        tunnel: [w248] -> w194
                        tunnel: w195 -> [w247]
                        tunnel: [w247] -> w193
                        tunnel: w190 -> [w246]
                        tunnel: w189 -> [w245]
                        tunnel: [w244] -> w192
                        tunnel: [w243] -> w191
                        tunnel: [w238] -> w178
                        tunnel: w177 -> [w238]
                        tunnel: w194 -> [w352]
                        tunnel: [w350] -> w187
                        tunnel: w193 -> [w349]
                        tunnel: [w348] -> w185
                        tunnel: [w347] -> w179
                        tunnel: w178 -> [w347]
                        tunnel: w187 -> [w404]
                        tunnel: [w404] -> w186
                        tunnel: w185 -> [w403]
                        tunnel: [w403] -> w184
                        tunnel: w183 -> [w400]
                        tunnel: w182 -> [w399]
                        tunnel: w181 -> [w398]
                        tunnel: w179 -> [w397]
                        tunnel: [w395] -> w176
                        tunnel: [w394] -> w174
                        tunnel: [w452] -> w202
                        tunnel: w186 -> [w452]
                        tunnel: [w451] -> w200
                        tunnel: w184 -> [w451]
                        tunnel: w176 -> [w450]
                        tunnel: [w450] -> w175
                        tunnel: w174 -> [w448]
                        tunnel: w173 -> [w449]
                        frame #0 {
                          # "Run Scan: Rotate half-wave plate to move piezo"
                          n73 = local read "Run Scan"() -> (w208:bool)
                          n74 = case shown="True" w208 {
                            tunnel: w205 -> [_ w209]
                            frame False {
                            }
                            frame True {
                              n75 = flat-sequence {
                                tunnel: [w217] -> w212
                                tunnel: [w214] -> w211
                                tunnel: w212 -> [w232]
                                tunnel: w211 -> [w233]
                                tunnel: [w232] -> w210
                                tunnel: w209 -> [w221]
                                tunnel: w210 -> [w235]
                                frame #0 {
                                n76 = local read "StepNb"() -> (w214:i32)
                                n77 = Increment(x=w214) -> (x+1=w213:i32)
                                n78 = Increment(x=w214) -> (x+1=w218:i32)
                                n79 = Equal?(x=w218, y="Max Steps") -> (x = y?=→"End of scan":bool)
                                n80 = Less?(x=w213, y="Max Steps") -> (x < y?=w217:bool)
                                n81 = local write "Run Scan"(w217) -> ()
                                }
                                frame #1 {
                                n82 = node(ext[unit] 299792458.0) -> (w228:ext)
                                n83 = Multiply(x="Step (fs)", y=w233) -> (x*y=w231:dbl)
                                n84 = Add(x=w231, y="Start Delay (fs)") -> (x+y=w226:dbl)
                                "Current Delay (fs)" <- w226
                                n85 = Compound Arithmetic op=MULTIPLY(w226, w228, ext 360.0 ("y")) -> (w220:ext)
                                n86 = Divide(x=w220, y=ext 2128.0) -> (x/y=w222:ext)
                                "Angle [deg]" <- w222
                                n87 = call <userlib>:"CONEX-CC Absolute Move v2.vi"("Target position"=w222, "Connection Cluster in"=w221) -> ("Connection Cluster out"=w225:T8)  [unwired: 7 in]
                                n88 = call <userlib>:"Wait READY status.vi"("Connection Cluster in"=w225) -> ("Connection Cluster out"=w224:T8)  [unwired: 9 in, 1 out]
                                n89 = call <userlib>:"CONEX-CC Get Current Position v2.vi"("Connection Cluster in"=w224) -> ("Current position"=→"Current angle":dbl)  [unwired: 8 in, 2 out]
                                }
                                frame #2 {
                                n90 = case shown="True" w235 {
                                frame False {
                                }
                                frame True {
                                n91 = local read "StepNb"() -> (w237:i32)
                                n92 = Increment(x=w237) -> (x+1=w236:i32)
                                n93 = local write "StepNb"(w236) -> ()
                                }
                                }
                                }
                              }
                            }
                          }
                        }
                        frame #1 {
                          w252 = u16 1 items=["Stop", "Run"] ("RecordingState")
                          w249 = u16 0 items=["Stop", "Run"] ("RecordingState")
                          # "Check if recording is stopped"
                          # "Start recording"
                          # "Stop recording"
                          # "Take picture"
                          n94 = local read "Image buffer"() -> (w242:u64[])
                          n95 = local read "Nb of shot"() -> (w240:i32)
                          n96 = local write "Buffer0"(TRUE) -> ()
                          n97 = local write "Buffer1"(TRUE) -> ()
                          n98 = call "SetRecordingState.vi"("ErrorIn"=w245, "RecordingState"=w252, "ph"=w246) -> ("ErrorOut"=w260:errorcluster, "hout"=w259:u64)  [unwired: 2 in, 1 out]
                          n99 = flat-sequence {
                            tunnel: [w274] -> w265
                            tunnel: [w273] -> w264
                            tunnel: [w270] -> w263
                            tunnel: [w269] -> w262
                            tunnel: [w268] -> w261
                            tunnel: w259 -> [w272]
                            tunnel: w260 -> [w271]
                            tunnel: w242 -> [w266]
                            tunnel: w240 -> [w267]
                            tunnel: w265 -> [w340]
                            tunnel: w264 -> [w339]
                            tunnel: w263 -> [w337]
                            tunnel: w262 -> [w336]
                            tunnel: w261 -> [w338]
                            tunnel: [w340] -> w258
                            tunnel: [w339] -> w257
                            tunnel: [w335] -> w241
                            frame #0 {
                              n100 = for {
                                N: w267 -> [_]
                                tunnel: [w280] -> w270
                                tunnel: [w279] -> w269
                                tunnel: w272 -> [w287]
                                tunnel: [w300] -> w273
                                tunnel: w271 -> [w286]
                                tunnel: [w301] -> w274
                                tunnel: w266 -> [w299]
                                shift-right: [w275] -> w268
                                shift-left: w266 -> [w277]
                                i -> [w276]
                                # "Take the number of shots"
                                n101 = local read "BufNr0"() -> (w282:i16)
                                n102 = local read "BufNr1"() -> (w281:i16)
                                n103 = local read "Bits/pixel"() -> (w283:u16)
                                n104 = local read "YResAct"() -> (w280:u16)
                                n105 = call "ForceTrigger.vi"("ph"=w287, "error in (no error)"=w286) -> ("hout"=w284:u64, "error out"=w285:errorcluster)  [unwired: 1 in, 2 out]
                                n106 = local read "XResAct"() -> (w279:u16)
                                n107 = local read "Buffer0"() -> (w296:bool)
                                n108 = case shown="True" w296 {
                                tunnel: [w303 w312] -> w297
                                tunnel: [w302 w311] -> w298
                                tunnel: w282 -> [_ w304]
                                tunnel: w284 -> [w302 w310]
                                tunnel: w283 -> [_ w308]
                                tunnel: w279 -> [_ w307]
                                tunnel: w280 -> [_ w306]
                                tunnel: w285 -> [w303 w305]
                                frame False {
                                }
                                frame True {
                                w309 = i16 0
                                n109 = call "AddBufferEX.vi"("ph"=w310, "BuffNr"=w304, "1stImage"=w309, "LastImage"=w309, "error in (no error)"=w305, "XRes"=w307, "YRes"=w306, "BitPerPixel"=w308) -> ("hout"=w311:u64, "error out"=w312:errorcluster)  [unwired: 5 in, 1 out]
                                }
                                }
                                n110 = local read "Buffer1"() -> (w295:bool)
                                n111 = case shown="True" w295 {
                                tunnel: [w313 w323] -> w291
                                tunnel: [w314 w322] -> w292
                                tunnel: w281 -> [_ w321]
                                tunnel: w298 -> [w314 w320]
                                tunnel: w283 -> [_ w318]
                                tunnel: w279 -> [_ w317]
                                tunnel: w280 -> [_ w316]
                                tunnel: w297 -> [w313 w315]
                                frame False {
                                }
                                frame True {
                                w319 = i16 0
                                n112 = call "AddBufferEX.vi"("ph"=w320, "BuffNr"=w321, "1stImage"=w319, "LastImage"=w319, "error in (no error)"=w315, "XRes"=w317, "YRes"=w316, "BitPerPixel"=w318) -> ("hout"=w322:u64, "error out"=w323:errorcluster)  [unwired: 5 in, 1 out]
                                }
                                }
                                n113 = while {
                                tunnel: w282 -> [w331]
                                tunnel: w281 -> [w330]
                                tunnel: w292 -> [w333]
                                tunnel: w291 -> [w332]
                                tunnel: [w329] -> w290
                                tunnel: [w325] -> w288
                                tunnel: [w328] -> w289
                                stop <- w334 stop-if-true
                                # "Check for a buffer event to indicate an image is available"
                                n114 = call "WaitForBuffer.vi"("ph"=w333, "sBufNr"=w331, "sBufNr 2"=w330, "timeout"=5000, "error in (no error)"=w332) -> ("hout"=w329:u64, "Buffer_Ready"=w328:bool, "Buffer_Ready 2"=w327:bool, "error out"=w325:errorcluster)  [unwired: 10 in, 1 out]
                                n115 = Unbundle By Name(w325) -> ("status"=w324:bool)
                                n116 = Compound Arithmetic op=OR(w328, w327, w324) -> (w334:bool)
                                }
                                n117 = Not(x=w289) -> (.not. x?=w293:bool)
                                n118 = Select(t=w282, s=w289, f=w281) -> (s? t:f=w294:i16)
                                n119 = local write "Buffer0"(w289) -> ()
                                n120 = local write "Buffer1"(w293) -> ()
                                n121 = call "GetImageBuffer.vi"("ph"=w290, "BuffIn"=w299, "BuffNr"=w294, "error in (no error)"=w288, "xRes"=w279, "yRes"=w280, "Bitresolution"=w283) -> ("hout"=w300:u64, "BuffOut"=w278:u16[], "error out"=w301:errorcluster)  [unwired: 5 in, 1 out]
                                n122 = Add(x=w277, y=w278) -> (x+y=w275:u64[])
                                "Count" <- w276
                              }
                            }
                            frame #1 {
                              n123 = Reshape Array(w338, w337, w336) -> (w335:u64[][])
                            }
                          }
                          n124 = call "CancelImages.vi"("error in (no error)"=w258, "ph"=w257) -> ("error out"=w255:errorcluster, "hout"=w256:u64)  [unwired: 1 in, 1 out]
                          n125 = Divide(x=w241, y=w240) -> (x/y=→"CCD IMAGE":dbl[][])
                          n126 = call "SetRecordingState.vi"("ErrorIn"=w255, "RecordingState"=w249, "ph"=w256) -> ("ErrorOut"=w251:errorcluster, "hout"=w250:u64)  [unwired: 2 in, 1 out]
                          n127 = while {
                            tunnel: [w344] -> w244
                            tunnel: w251 -> [w345]
                            tunnel: w250 -> [w346]
                            tunnel: [w341] -> w243
                            stop <- w342 continue-if-true
                            n128 = call "GetRecordingState.vi"("ErrorIn"=w345, "ph"=w346) -> ("ErrorOut"=w344:errorcluster, "RecordingState"=w343:u16, "hout"=w341:u64)  [unwired: 2 in, 1 out]
                            n129 = Not Equal To 0?(x=w343) -> (x != 0?=w342:bool)
                          }
                          n130 = call <vilib>:"Simple Error Handler.vi"("error in (no error)"=w244) -> ()  [unwired: 4 in, 5 out]
                        }
                        frame #2 {
                          n131 = case shown="True" "Analyze" {
                            tunnel: w352 -> [w354 w381]
                            tunnel: [w354 w368] -> w350
                            tunnel: w349 -> [w353 w377]
                            tunnel: [w353 w367] -> w348
                            frame False {
                            }
                            frame True {
                              # "Analysis"
                              n132 = property on="Angle Integrated Spectrum" class="XYGraph (strict)"() -> ("CrsrList"=w384:T12)  [unwired: 2 in, 2 out]
                              n133 = Index Array(array=w384, index #1=0, index #2=1) -> (element #1=w366:T13, element #2=w365:T13)
                              n134 = Unbundle By Name(w366) -> ("Position.X"=w364:dbl)
                              n135 = Unbundle By Name(w365) -> ("Position.X"=w363:dbl)
                              n136 = Bundle By Name(cluster="Area Parameteres", "Center angle (deg)"="Center angle (deg)", "Arc length (deg)"="Arc length (deg)", "Angle step (deg)"="Angle step (deg)", "Outer radius"="Outer radius", "Inner radius"="Inner radius", "Radius"=0.0 ("Arc length (deg)"), "Radial step"="Radial step") -> (w378:T2)
                              n137 = property on="CCD IMAGE" class="IntGraph (strict)"() -> ("Cursor.Cursor Position:Cursor X"=w380:dbl, "Cursor.Cursor Position:Cursor Y"=w379:dbl)  [unwired: 2 in, 2 out]
                              n138 = local read "CCD IMAGE"() -> (w382:dbl[][])
                              n139 = Build Array(w380, w379) -> (w362:dbl[])
                              n140 = Build Array(w364, w363) -> (w361:dbl[])
                              n141 = call "Analysis.vi"("CCD image"=w382, "CCD image Cursor position"=w362, "Angle integrated Cursor position"=w361, "Area Parameters"=w378, "Energy/Radius"="Energy/Radius", "index (row)"="index (row)", "Spec Up"=w381, "Spec Down"=w377) -> ("Picture"=→"Picture":cluster{dbl[], dbl[]}[], "Angular distribution"=→"Angular distribution":dbl[][], "Angular distribution 2"=→"Angular distribution 2":dbl[][], "Spectrogram Up"=w368:dbl[][], "Spectrogram Down"=w367:dbl[][], "Angle Integrated Spectrum"=→"Angle Integrated Spectrum":T5, "Fully Integrated Spectrum"=→"Fully Integrated Spectrum":dbl, "Angle Integrated Spectrum 2"=→"Angle Integrated Spectrum 2":T1, "Range scan"=w359:dbl[][], "Asymetry Spectrogram"=→"Asymetry spectrogarm":dbl[][])  [unwired: 1 in, 1 out]
                              "Range scan" <- w359
                              "Spectrogram up" <- w368
                              "Spectrogram down" <- w367
                              n142 = Index Array(array=w359, index (row)=0) -> (element=w357:dbl[])  [unwired: 1 in]
                              n143 = call-poly <vilib>:"FFT.vi"("X"=w357) -> ("FFT {X}"=w356:cdb[])  [unwired: 9 in, 1 out]
                              n144 = Complex To Polar(r * e^(i*theta)=w356) -> (r=→"FFT":dbl[])  [unwired: 1 out]
                            }
                          }
                        }
                        frame #3 {
                          n145 = flat-sequence {
                            tunnel: [w409] -> w402
                            tunnel: w400 -> [w406]
                            tunnel: w399 -> [w405]
                            tunnel: w402 -> [w414]
                            tunnel: [w414] -> w401
                            tunnel: w401 -> [w424]
                            tunnel: [w424] -> _
                            tunnel: w398 -> [w423]
                            tunnel: [w422] -> w396
                            tunnel: [w421] -> w394
                            frame #0 {
                              n146 = case shown="True" w405 {
                                tunnel: [FALSE w413] -> w409
                                tunnel: w406 -> [_ w411]
                                frame False {
                                }
                                frame True {
                                n147 = dll-call lib="atmcd32d.dll" fn="StartAcquisition" label="Call Library Function start acquisition"() -> (w412:u32)  [unwired: 3 in, 2 out]
                                "Start Acquisition" <- w412
                                n148 = Equal?(x=w412, y=w411) -> (x = y?=w413:bool)
                                }
                              }
                              n149 = property on="Camera Status:" class="Bool (strict)"("BoolText.Text"="Running..." ("Boolean Text.Text")) -> ()  [unwired: 2 in, 2 out]
                              n150 = local write "Camera Status:"(TRUE ("Camera Status:")) -> ()
                            }
                            frame #1 {
                              n151 = case shown="True" w414 {
                                frame False {
                                }
                                frame True {
                                n152 = while {
                                stop <- w418 continue-if-true
                                w417 = u16 20072  # DRV ACQUIRING
                                n153 = dll-call lib="atmcd32d.dll" fn="GetStatus" label="Call Library Function GetAcquisitionStatus"(u16 0) -> (→"Get Status":u32, w416:u32)  [unwired: 3 in, 2 out]
                                "Status" <- w416
                                n154 = Wait Until Next ms Multiple "Wait"(millisecond multiple=u32 250) -> ()  [unwired: 1 out]
                                n155 = Equal?(x=w416, y=w417) -> (x = y?=w418:bool)
                                }
                                }
                              }
                            }
                            frame #2 {
                              n156 = case shown="True" w423 {
                                tunnel: [_ w428] -> w421
                                tunnel: [_ w425] -> w422
                                frame False {
                                }
                                frame True {
                                n157 = local read "Detector Y Pixels"() -> (w434:i32)
                                n158 = local read "Detector X Pixels"() -> (w430:i32)
                                n159 = Multiply(x=w434, y=w430) -> (x*y=w436:i32)
                                n160 = Initialize Array "Initialize Array"(0 ("Initial values in array"), w436) -> (w438:i32[])
                                n161 = To Long Integer(number=w436) -> (32bit integer=w437:i32)
                                n162 = dll-call lib="atmcd32d.dll" fn="GetAcquiredData" label="Call Library Function Get Acquired data"(w438, w437) -> (→"Get Acquired Data":u32, w435:i32[])  [unwired: 4 in, 2 out]
                                n163 = Reshape Array(w435, w434, w430) -> (w428:i32[][])
                                n164 = call "Imageflip.vi"("2D array"=w428) -> ("transposed array"=w427:i32[][])
                                "Raw Image" <- w427
                                n165 = Transpose 2D Array(2D array=w427) -> (transposed array=w433:i32[][])
                                n166 = Array Max & Min(array=w427) -> (max value=w432:i32)  [unwired: 3 out]
                                n167 = for {
                                tunnel: w433 -> [w447] mode=indexing
                                tunnel: [w446] -> w425 mode=indexing
                                n168 = Add Array Elements(numeric array=w447) -> (sum=w446:i32)
                                }
                                "VBI" <- w425
                                n169 = Greater?(x=w432, y=64900) -> (0:w431:bool)
                                n170 = case shown="True" w431 {
                                frame False {
                                }
                                frame True {
                                n171 = local write "Camera Status:"(FALSE ("Camera Status:")) -> ()
                                n172 = property on="Camera Status:" class="Bool (strict)"("BoolText.Text"="Saturated!" ("Boolean Text.Text")) -> ()  [unwired: 2 in, 2 out]
                                n173 = Two Button Dialog(message="Camera is saturating! Reduce photon flux!", 1:"I've fixed it, and I want to continue" ("message"), 2:"Shut Down acquisition program" ("T button name (\"OK\")")) -> (T button?=w440:bool)
                                n174 = local write "Stop"(w440) -> ()
                                n175 = local write "Exit"(w440) -> ()
                                }
                                }
                                }
                              }
                            }
                          }
                          n176 = Insert Into Array(array=w397, new element=w396) -> (w395:dbl[][])  [unwired: 2 in]
                          "XUV" <- w395
                        }
                        frame #4 {
                          # "Save image and delays"
                          n177 = case shown="True" "Save image" {
                            tunnel: w449 -> [_ w456]
                            tunnel: w448 -> [_ w454]
                            frame False {
                            }
                            frame True {
                              n178 = stacked-sequence {
                                frame #0 {
                                n179 = local read "Actual delay  (fs)"() -> (w462:dbl)
                                n180 = local read "CCD IMAGE"() -> (w461:dbl[][])
                                n181 = local read "Index"() -> (w460:i32)
                                n182 = call "Save Images and Delays.vi"("Delay [fs]"=w462, "Array"=w461, "Index"=w460, "Name"="Name", "Path"="Path") -> ()
                                }
                                frame #1 {
                                n183 = local read "Index"() -> (w464:i32)
                                n184 = Increment(x=w464) -> (x+1=w463:i32)
                                n185 = local write "Index"(w463) -> ()
                                }
                              }
                              n186 = Equal To 0?(x=w456) -> (x = 0?=w457:bool)
                              n187 = call "save image.vi"("Start of pump/prove run?"=w457, "Image to save"=w454, "Pump/probe run?"=TRUE) -> ()  [unwired: 1 out]
                            }
                          }
                        }
                      }
                      n188 = local read "End of scan"() -> (w197:bool)
                      n189 = Or(x=w197, y="Stop") -> (x .or. y?=w199:bool)
                    }
                  }
                  frame #2 {
                    w465 = FALSE ("Start Measurement")
                    # "Free up any allocated buffers and close the camera communication channel"
                    # "Quit:"
                    # "Set the start button to false"
                    n190 = call "Cleanup.vi"("error in (no error)"=w467, "ph"=w466) -> ("error out"=w469:errorcluster, "hout"=w470:u64)  [unwired: 8 in]
                    n191 = property on="Start Measurement" class="Bool (strict)"("Value"=w465) -> ()  [unwired: 2 in, 2 out]
                    n192 = local write "Start Measurement"(w465) -> ()
                    n193 = local write "Take image"(w465) -> ()
                    n194 = local write "Run Scan"(w465) -> ()
                    n195 = call "CloseCamera.vi"("ErrorIn"=w469, "Handle in"=w470) -> ("ErrorOut"=w471:errorcluster)  [unwired: 1 in, 2 out]
                    n196 = call <vilib>:"Simple Error Handler.vi"("error in (no error)"=w471) -> ()  [unwired: 4 in, 5 out]
                    n197 = One Button Dialog(message="Measurement completed!") -> ()  [unwired: 1 in, 1 out]
                  }
                }
              }
            }
          }
        }
      }
    }
    frame #3 {
      w474 = FALSE
      n198 = flat-sequence {
        tunnel: w472 -> [w481]
        tunnel: [w481] -> w473
        tunnel: w473 -> [w483]
        frame #0 {
          n199 = local write "Camera Status:"(FALSE ("Camera Status:")) -> ()
          n200 = property on="Camera Status:" class="Bool (strict)"("BoolText.Text"="Shutting Down..." ("Boolean Text.Text")) -> ()  [unwired: 2 in, 2 out]
        }
        frame #1 {
          n201 = call "ShutDownSubVI.vi"("shutdown"=w483) -> ("Shut Down"=→"Shut Down":u32)
        }
      }
      n202 = Unbundle By Name(w475) -> ("VISA resource name"=w478:refnum<visa-resource-name>, "error"=w477:errorcluster)
      n203 = local write "Connected"(w474) -> ()
      n204 = local write "Ready"(w474) -> ()
      n205 = call <userlib>:"_Close Communications.vi"("Instrument Channel"=w478, "error in (no error)"=w477) -> ("error out"=w476:errorcluster)  [unwired: 13 in]
      n206 = call <vilib>:"General Error Handler.vi"("error in (no error)"=w476) -> ()  [unwired: 10 in, 5 out]
    }
  }
